vi "op_EQ_wHV.vi"(0 "Addresses Cluster":T1={"ENA1"=FALSE, "IP address 1"="172.16.14.22", "ENA2"=FALSE, "IP address 2"="172.16.14.23"}, 2 "HV parameters":T3={"Final value"=-1000, "Number of steps"=10, "Time/step"=800, "Output Off Behavior"=0, "VISA resource name"="GPIB1::25::INSTR"} {"Output Off Behavior" items=["Normal", "High Impedance", "Zero", "Guard"]; "Time/step" min=100 max=2000 step=100; "Final value" min=-1100 max=0 step=10; "Number of steps" min=10 max=20 step=10}, 3 "HV level Refnum":refnum<vi>, 4 "HV string Refnum":refnum<vi>, 5 "error tick Refnum":refnum<vi>, 6 "Operation text Refnum":refnum<vi>, 7 "EQ timeout auto Refnum":refnum<vi>, 8 "EQ wHV step barra Refnum":refnum<vi>, 9 "etapa# terminals refnums":T2, 10 "Busy Refnum":refnum<vi>, 11 "EQ steps":bool, 12 "notifier crono/Ileak":refnum<notifier>, 13 "Stop subVI Refnum":refnum<vi>) -> (15 "Folder path: equalization reports":path=path "C:/VIP Module/Files/Equalization/yyyymmdd_hh-mm-ss_Leak#_HV#", 18 "IDs summary":string, 19 "EQ summary":string)   [LabVIEW 2015, in "VIPM2.lvlib"]
doc: "Uses Notifier for Start/Stop/Exit Crono per ordres separades.\nbusy = F while waiting times and HV ramps."
uses:
  VIPM2.lvlib
panel:
  out "quants Layer":i32
  out "Chip ID list 1i2":u32[](array[numeric]) format="%.0x"
  out "I Leak":u8=3 max=3 step=1
  out "Global Reg (hex)":u32[](array[numeric])=[68228136, 235670073, 4294967264, 4294967295, 4294967295, 511] format="%x"
  out "PixelReg (hex)":u32[](array[numeric])=[671965161, 384, 671965161, 384, 671965161, 384, 671965161, 384, 671965161, 384, 671965161, 384, 671965161, 384, 671965161, 384, 671965161, 384, 671965161, 384, 671965161, 384, 671965161, 384, 671965161, 384, 671965161, 384, 671965161, 384, 671965161, 384, 671965161, 384, 671965161, 384, 671965161, 384, 671965161, 384, 671965161, 384, 671965161, 384, 671965161, 384, 671965161, 384, 671965161, 384, 671965161, 384, 671965161, 384, 671965161, 384, 671965161, 384, 671965161, 384, 671965161, 384, 671965161, 384, 671965161, 384, 671965161, 384, 671965161, 384, 671965161, 384, 671965161, 384, 671965161, 384, 671965161, 384, 671965161, 384, 671965161, 384, 671965161, 384, 671965161, 384, 671965161, 384, 671965161, 384, 671965161, 384, 671965161, 384, 671965161, 384, 671965161, 384, 671965161, 384, 671965161, 384, 671965161, 384, 671965161, 384, 671965161, 384, 671965161, 384, 671965161, 384, 671965161, 384, 671965161, 384, 671965161, 384, 671965161, 384, 671965161, 384, 671965161, 384, 671965161, 384, 671965161, 384, 671965161, 384, 671965161, 384, 671965161, 384, 671965161, 384, 671965161, 384, 671965161, 384, 671965161, 384, 671965161, 384, 671965161, 384, 671965161, 384, 671965161, 384, 671965161, 384, 671965161, 384, 671965161, 384, 671965161, 384, 671965161, 384, 671965161, 384, 671965161, 384, 671965161, 384, 671965161, 384, 671965161, 384, 671965161, 384, 671965161, 384, 671965161, 384, 671965161, 384, 671965161, 384, 671965161, 384, 671965161, 384, 671965161, 384, 671965161, 384, 671965161, 384, 671965161, 384, 671965161, 384, 671965161, 384, 671965161, 384, 671965161, 384] format="%x"
  in  "EQ parameters (cluster)":T4={"Timeout ITEST sweep"=21, "Number pulses ITEST"=20, "TOT"=40, "ADC target"=900, "Number pulses SSpeak sweep"=100, "Timeout SSpeak sweep"=110, "Timeout THLD sweep"=10, "Number triggers THLD sweep"=2, "First PIXEL"=0, "Last PIXEL"=99, "Sigma factor"=2, "DTP period for SSpeak sweep"=1, "Global THR for ITEST sweep"=38, "Pulse width"=0} {"Number triggers THLD sweep" step=1; "Timeout THLD sweep" step=1; "Timeout SSpeak sweep" step=1; "DTP period for SSpeak sweep" step=1; "Number pulses SSpeak sweep" step=1; "Timeout ITEST sweep" step=1; "Global THR for ITEST sweep" step=1; "Number pulses ITEST" step=1; "Pulse width" items=["25 ns", "50 ns", "75 ns", "100 ns"]; "Sigma factor" step=1; "Last PIXEL" max=99 step=1; "First PIXEL" max=99 step=1; "ADC target" step=1; "TOT" step=1}
  # "Operation: EQualization with HV (refnums)"
  # "Uses Notifier for\nStart/Stop/Exit Crono"
  # "I test sweep"
  # "SS peak sweep"
  # "THLD sweep"
  # "Number of triggers"
  # "Timeout"
  # "Timeout"
  # "DTP period"
  # "Number of pulses"
  # "Timeout"
  # "Global THR"
  # "Number of pulses"
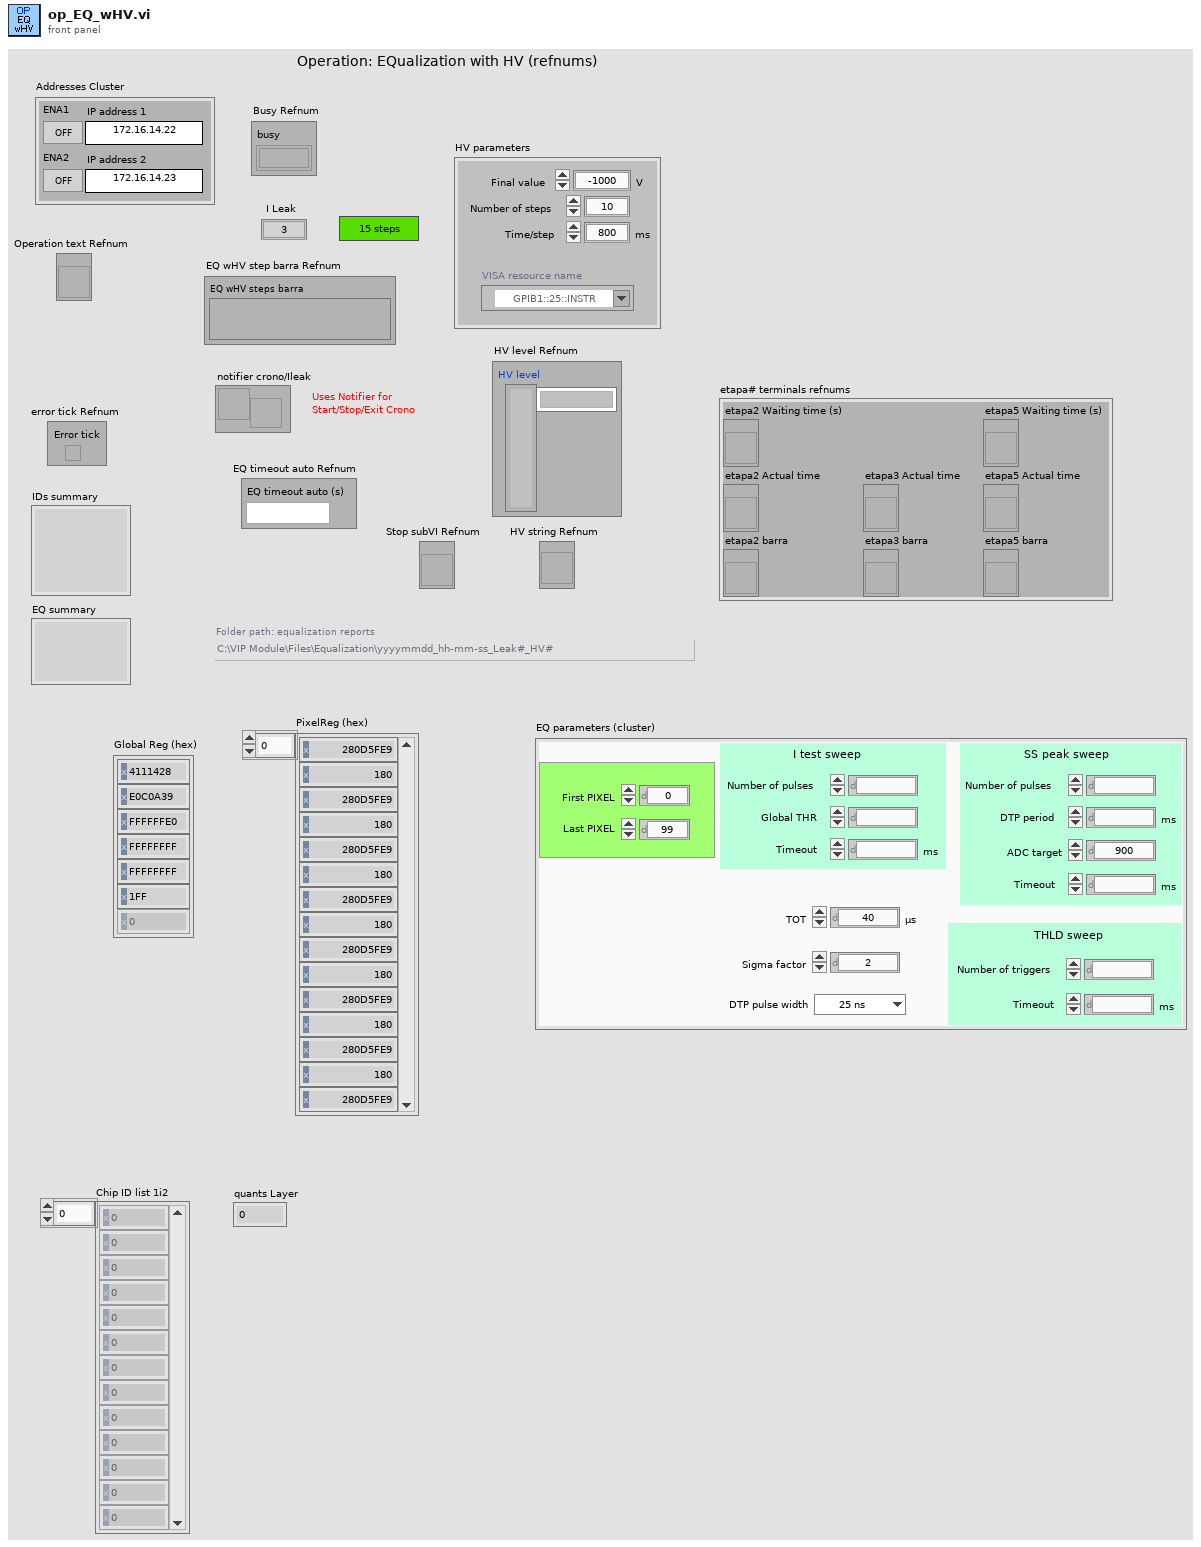
[diagram p1: front panel]
types:
  T1 = cluster{"ENA1":bool, "IP address 1":string, "ENA2":bool, "IP address 2":string}
  T2 = cluster{"etapa2 Waiting time (s)":refnum<vi>, "etapa2 Actual time":refnum<vi>, "etapa2 barra":refnum<vi>, "etapa3 Actual time":refnum<vi>, "etapa3 barra":refnum<vi>, "etapa5 Waiting time (s)":refnum<vi>, "etapa5 Actual time":refnum<vi>, "etapa5 barra":refnum<vi>}
  T3 = cluster{"Final value":i16, "Number of steps":u8, "Time/step":u16, "Output Off Behavior":u16, "VISA resource name":refnum<visa-resource-name>}
  T4 = cluster{"Timeout ITEST sweep":u32, "Number pulses ITEST":u32, "TOT":u32, "ADC target":u32, "Number pulses SSpeak sweep":u32, "Timeout SSpeak sweep":u32, "Timeout THLD sweep":u32, "Number triggers THLD sweep":u32, "First PIXEL":u32, "Last PIXEL":u32, "Sigma factor":u32, "DTP period for SSpeak sweep":u32, "Global THR for ITEST sweep":u32, "Pulse width":u32}
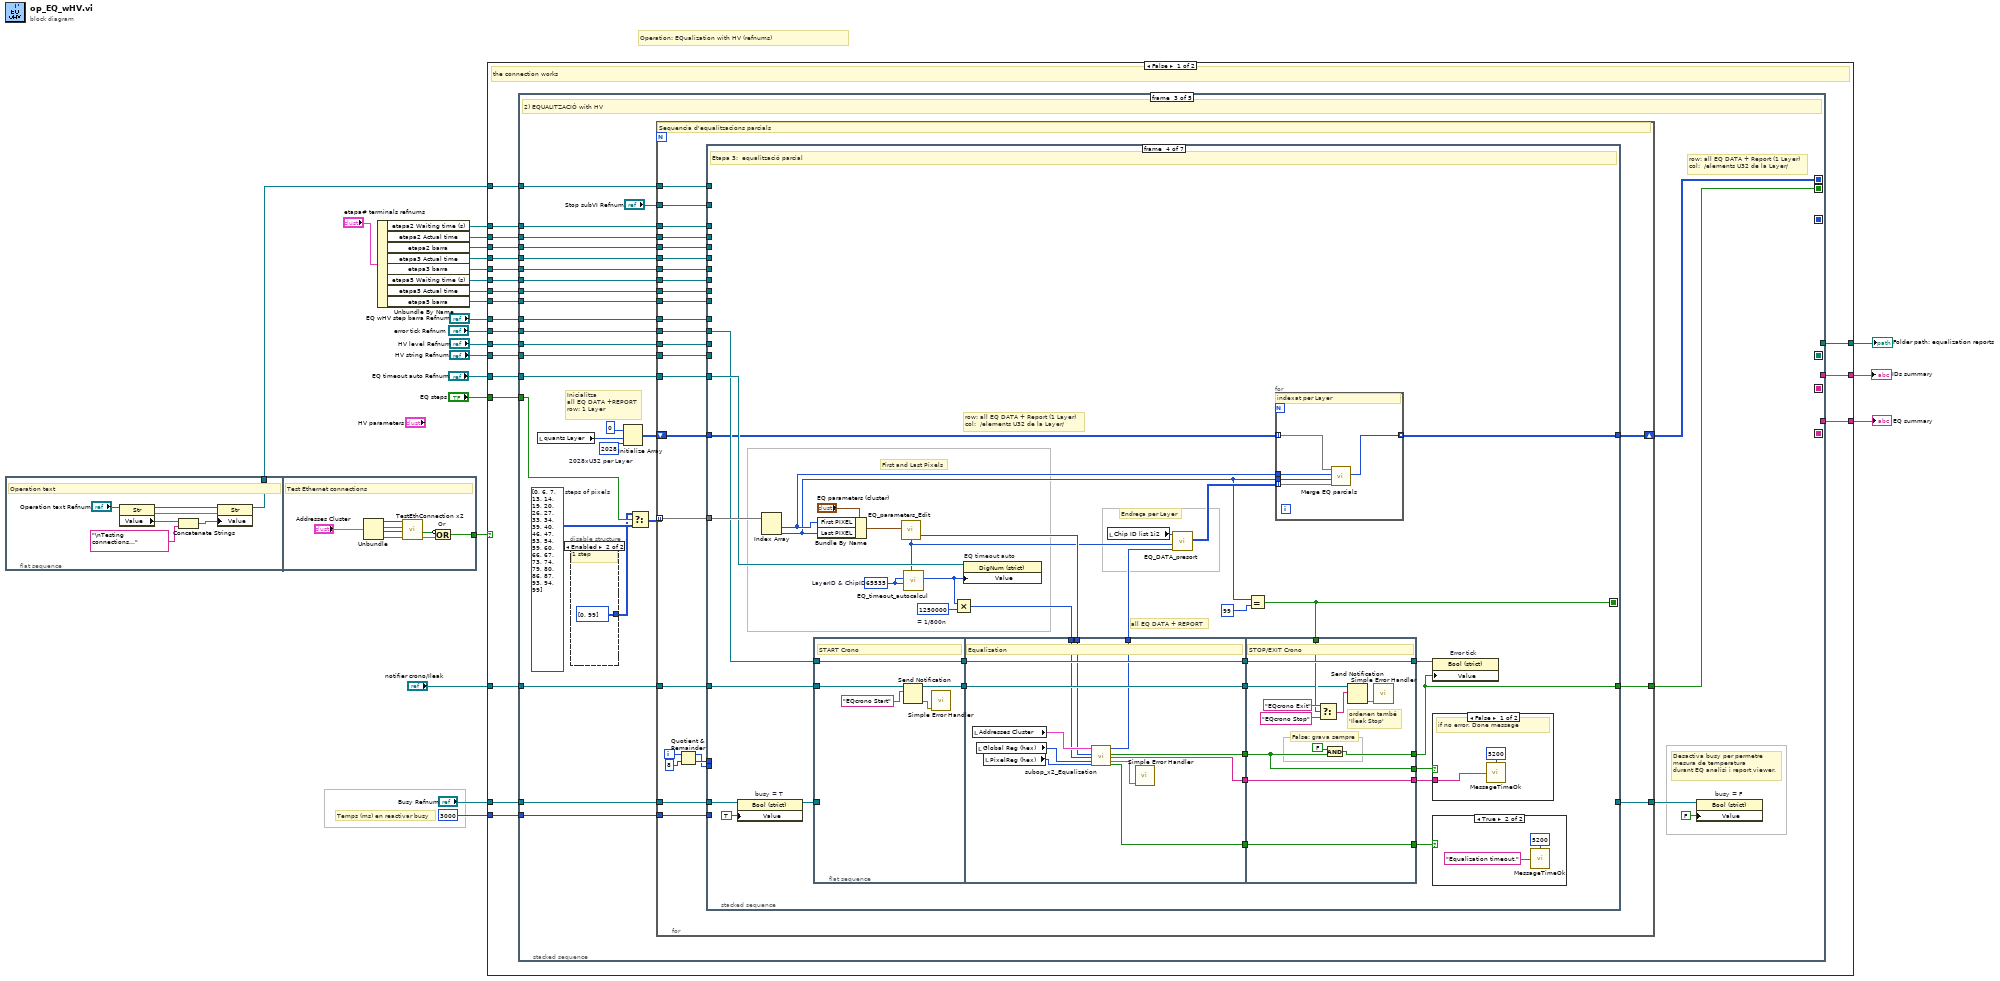
[diagram p0: block diagram]
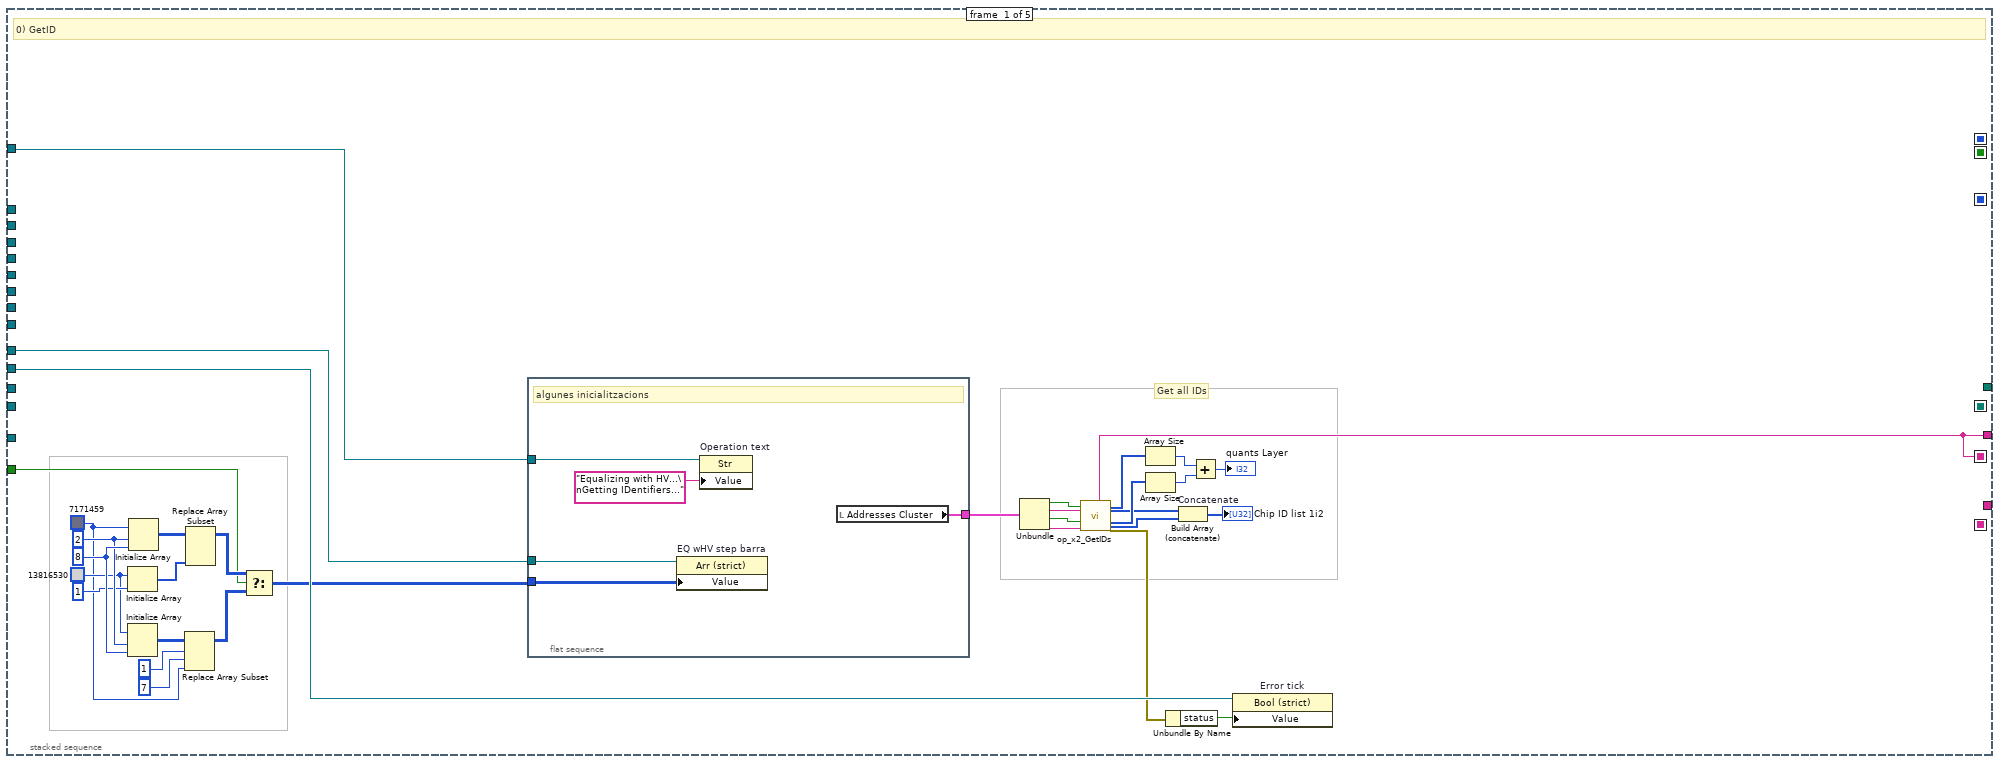
[diagram p2: hidden frame]
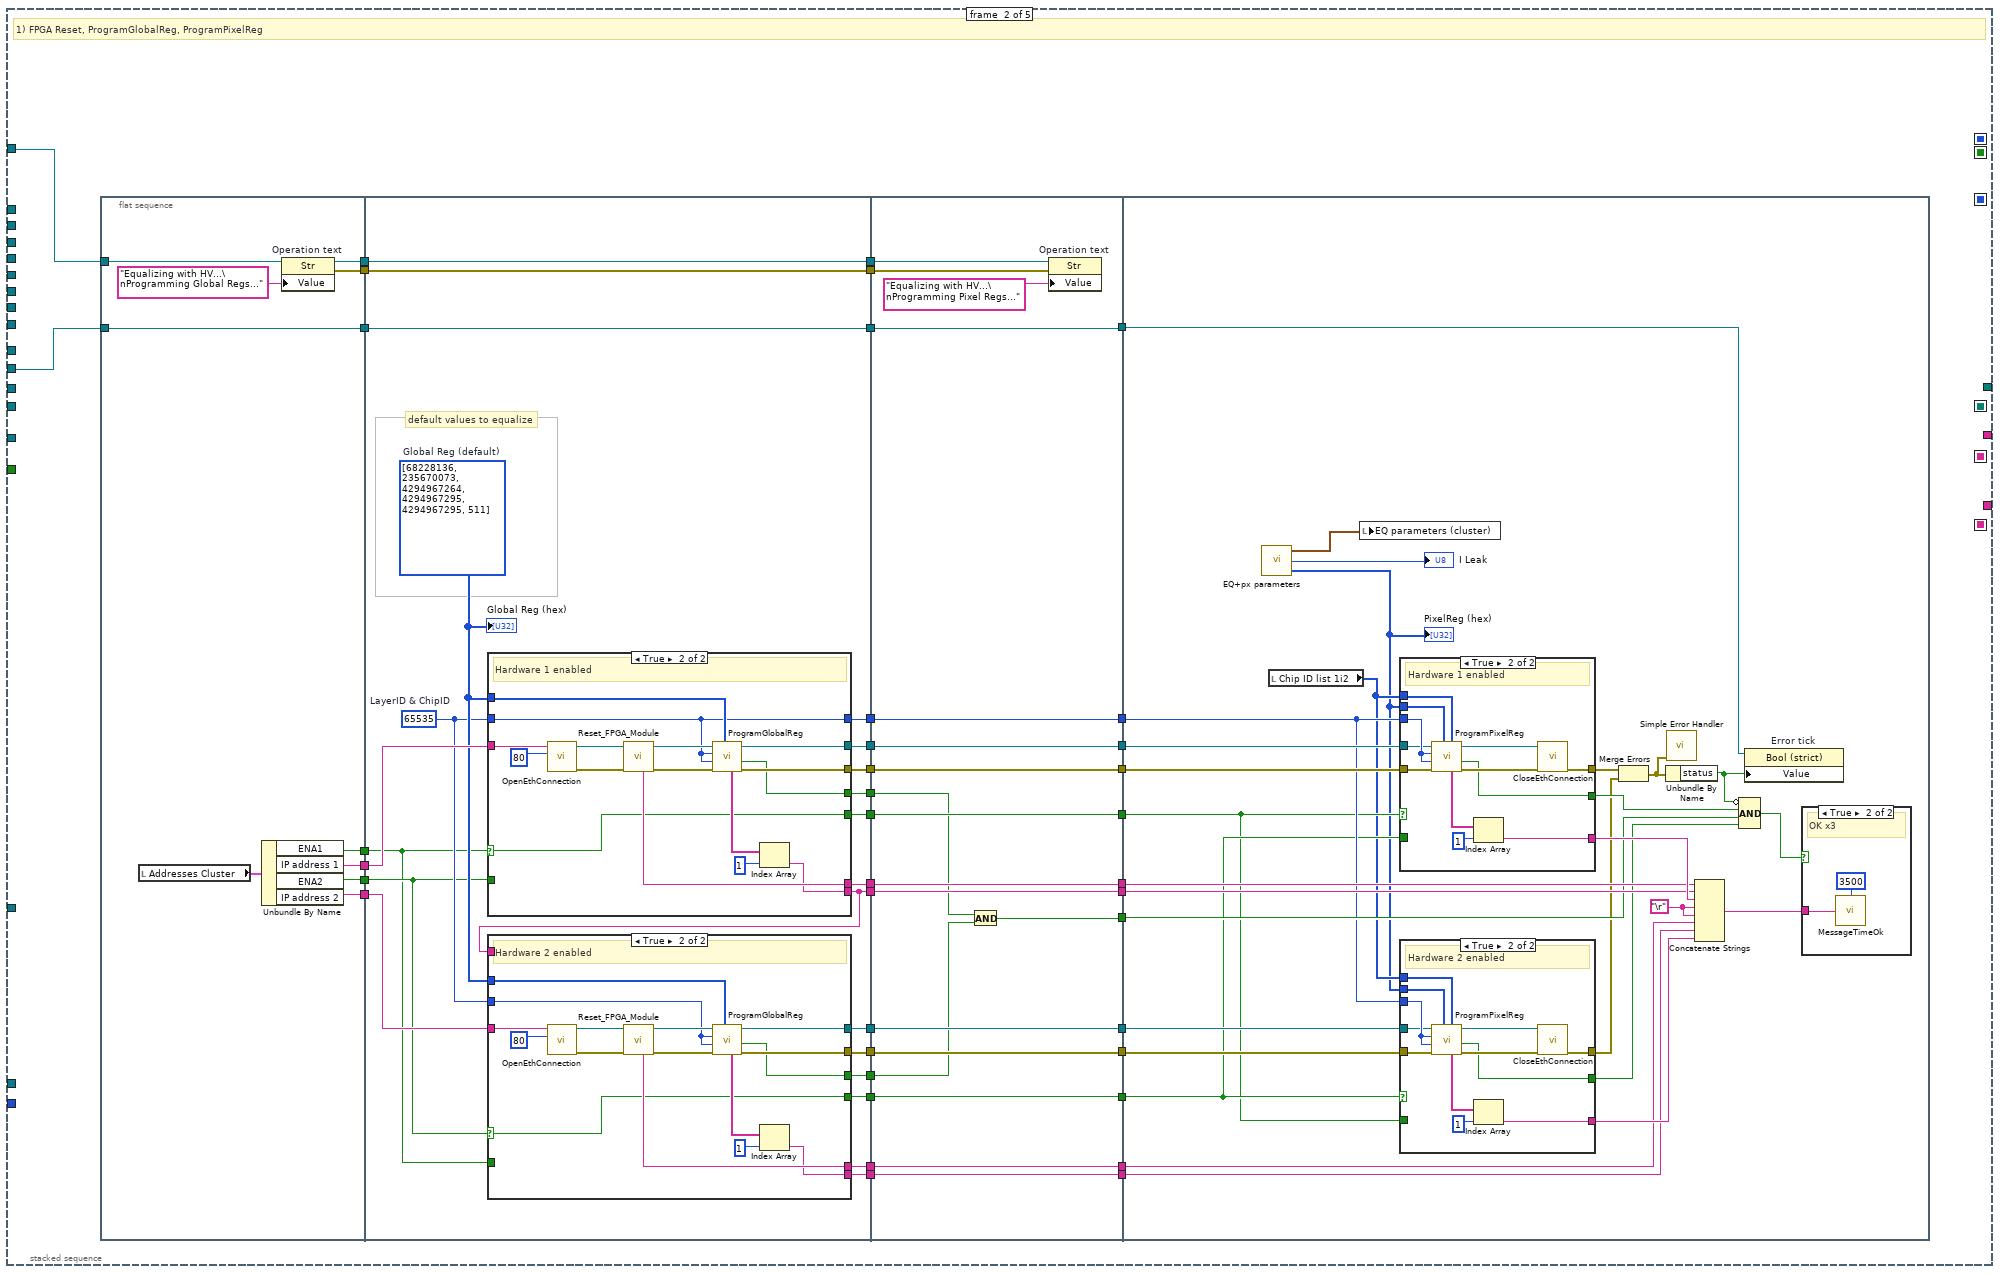
[diagram p3: hidden frame]
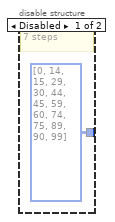
[diagram p9: hidden frame]
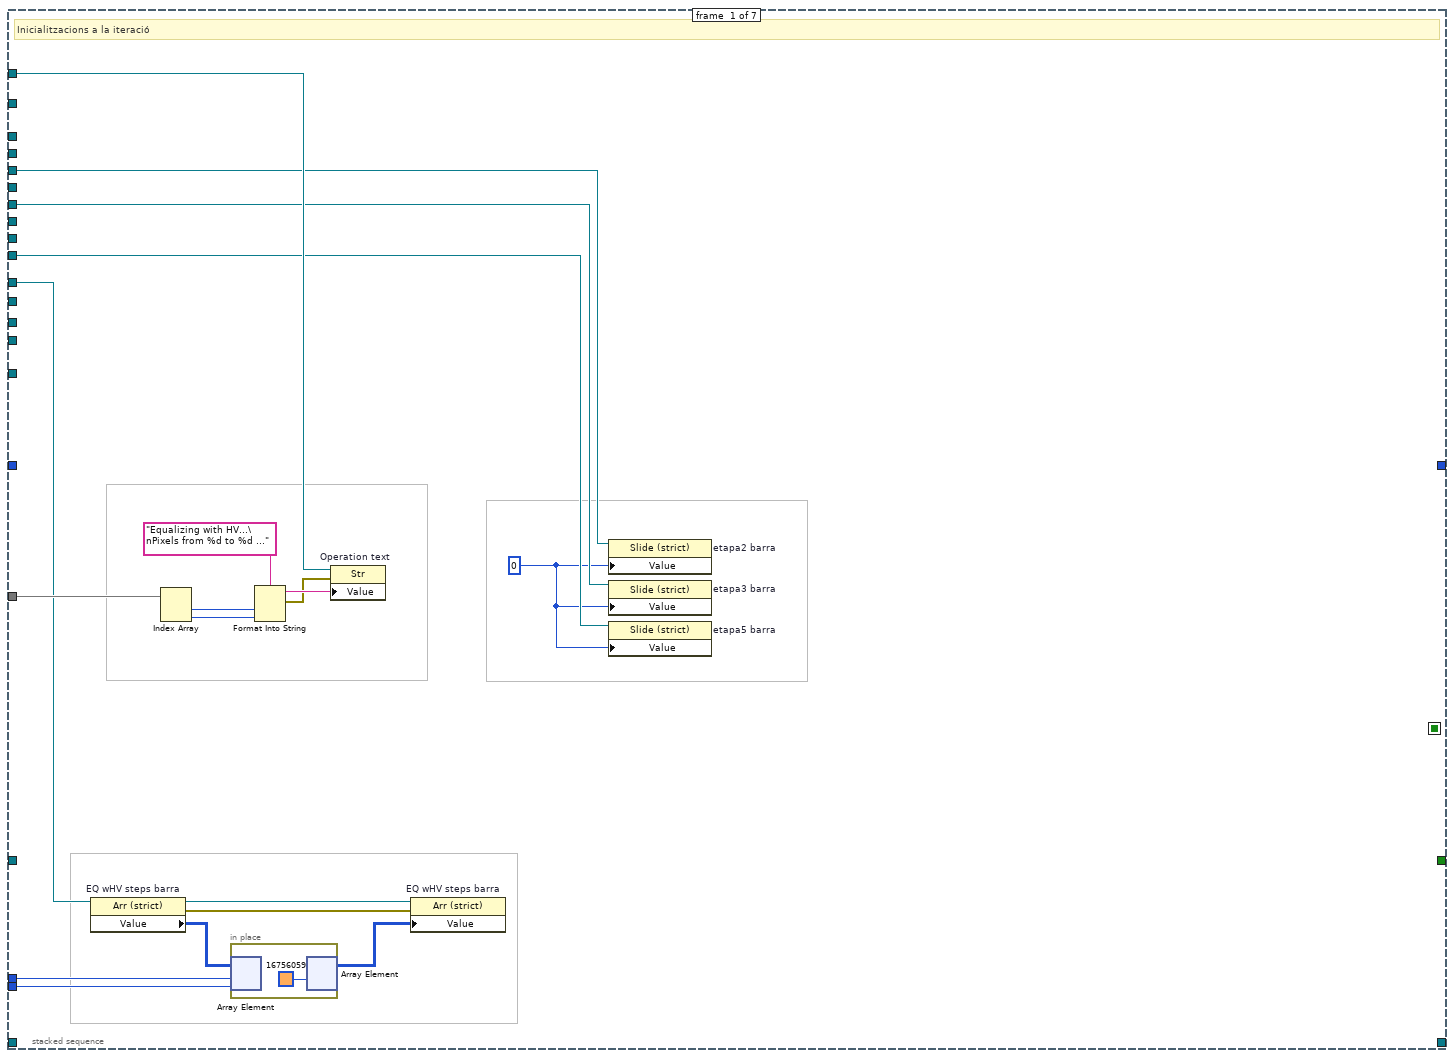
[diagram p10: hidden frame]
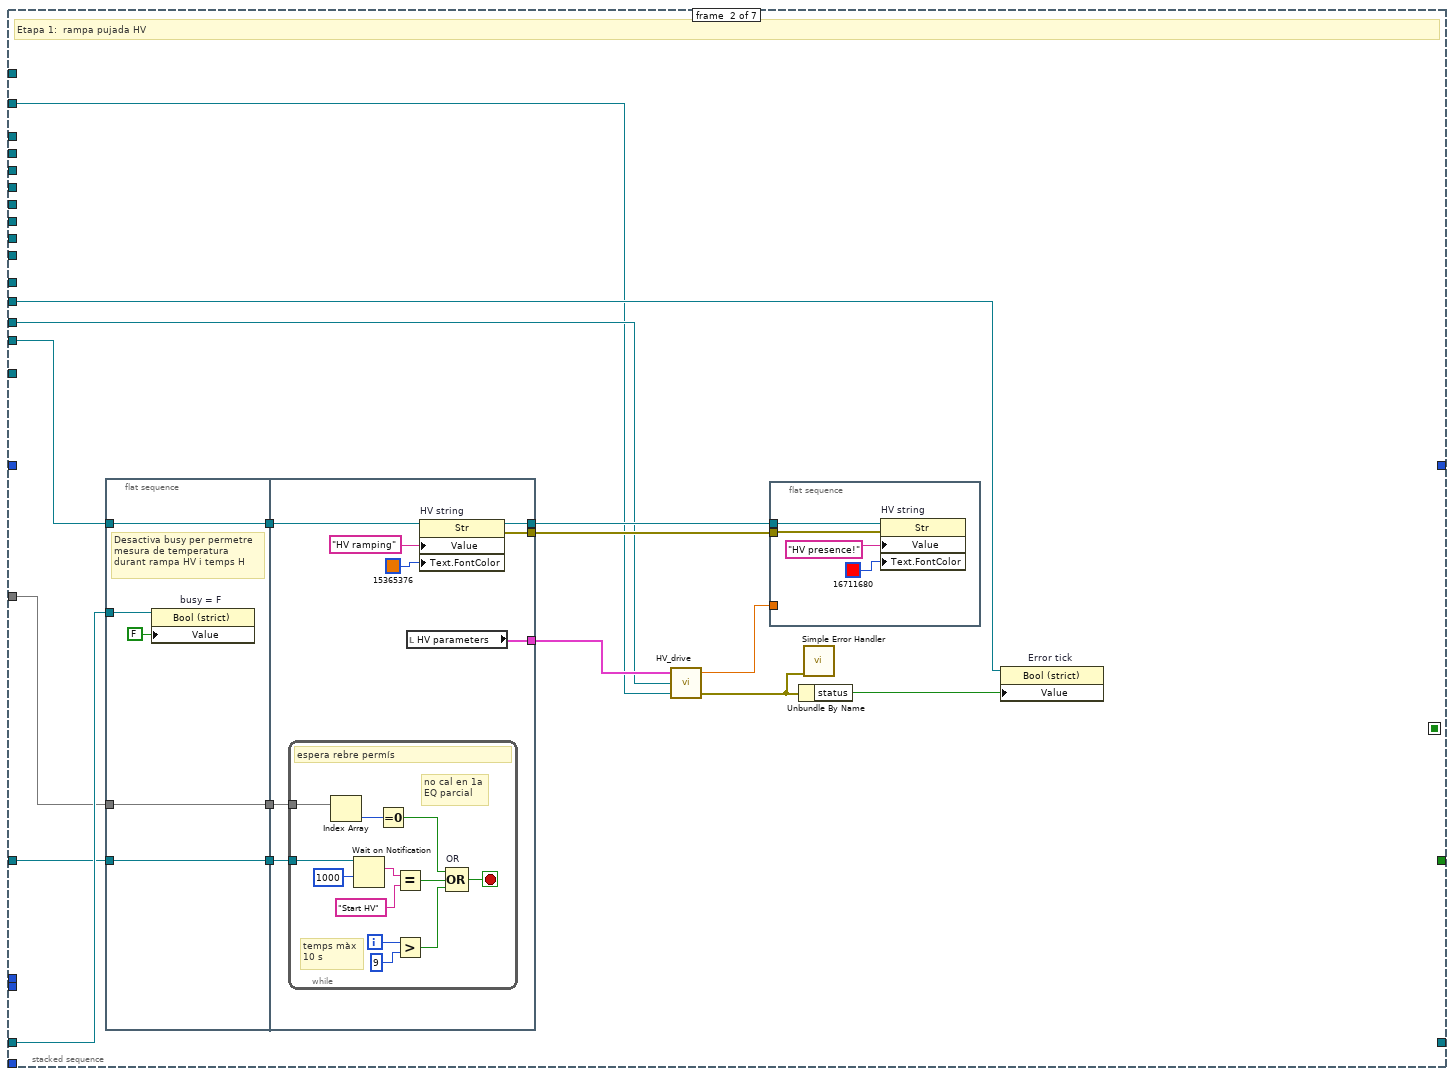
[diagram p11: hidden frame]
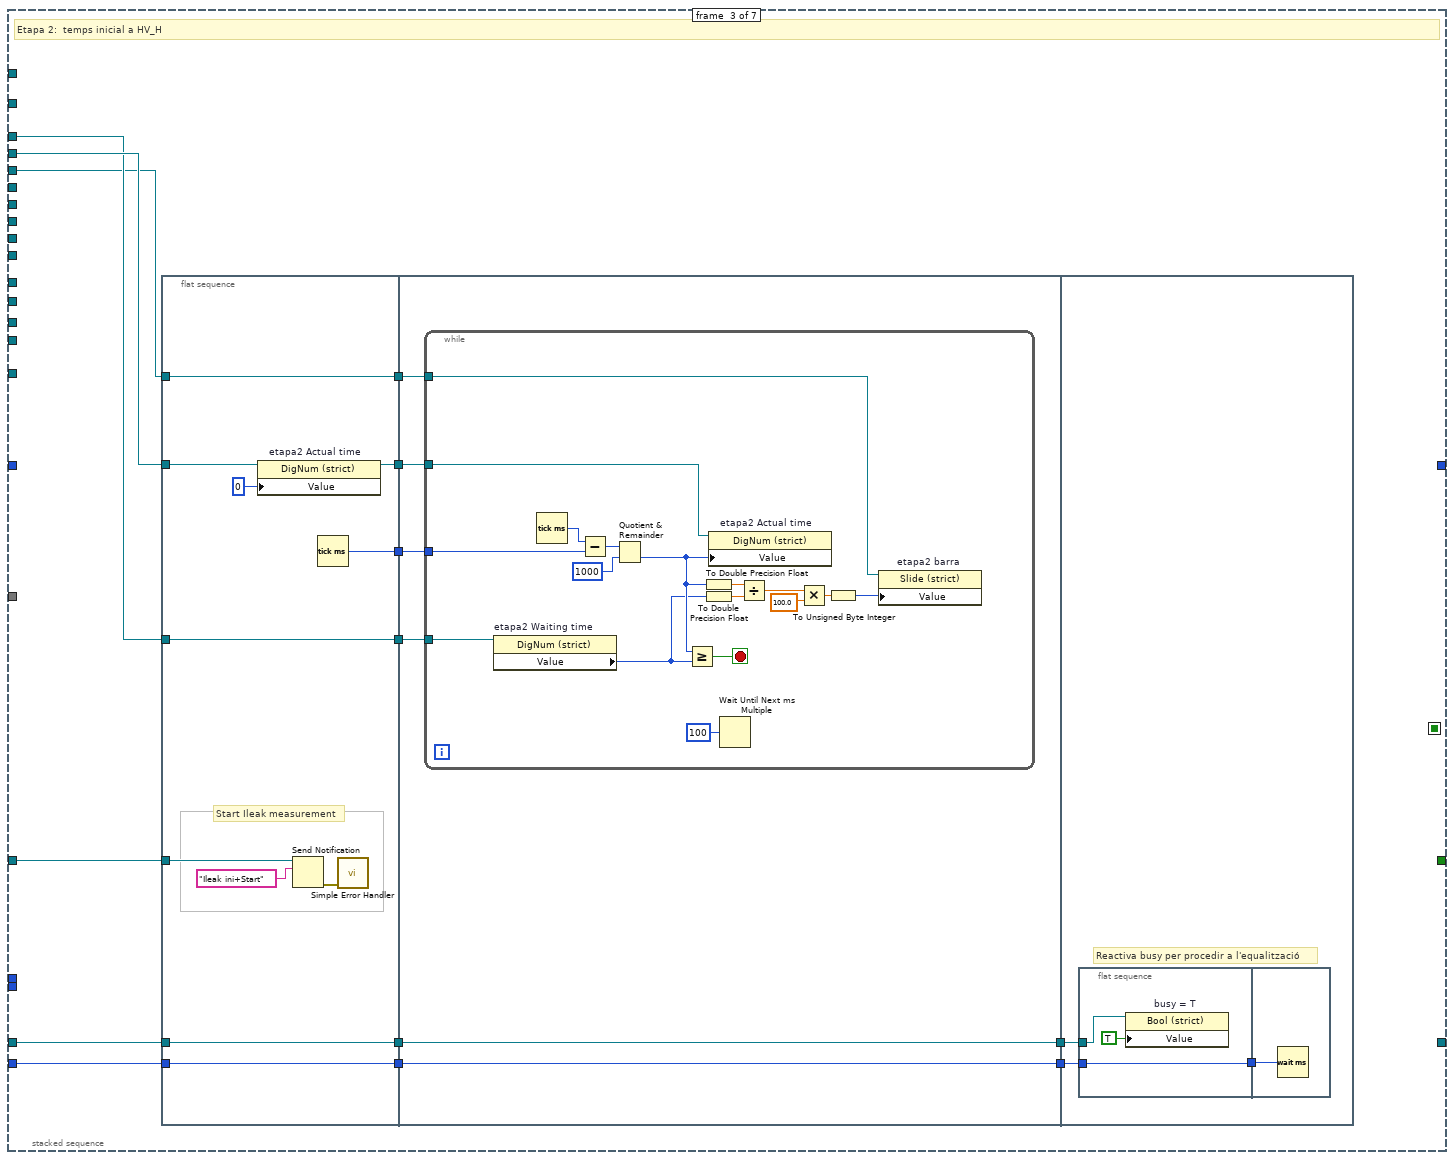
[diagram p12: hidden frame]
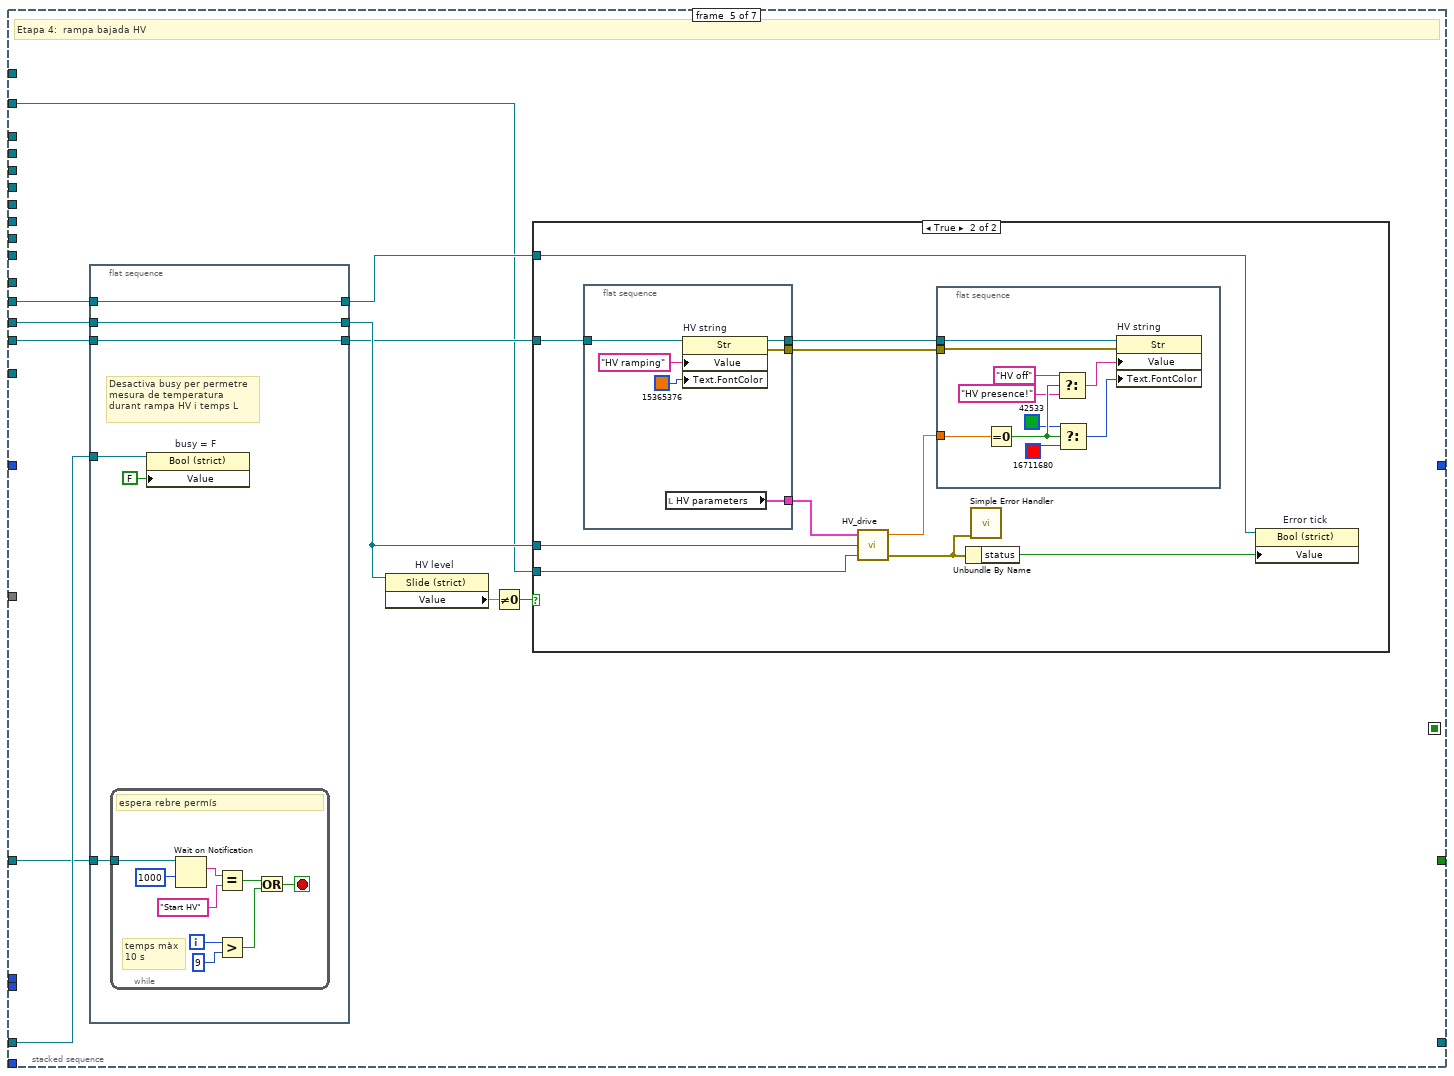
[diagram p15: hidden frame]
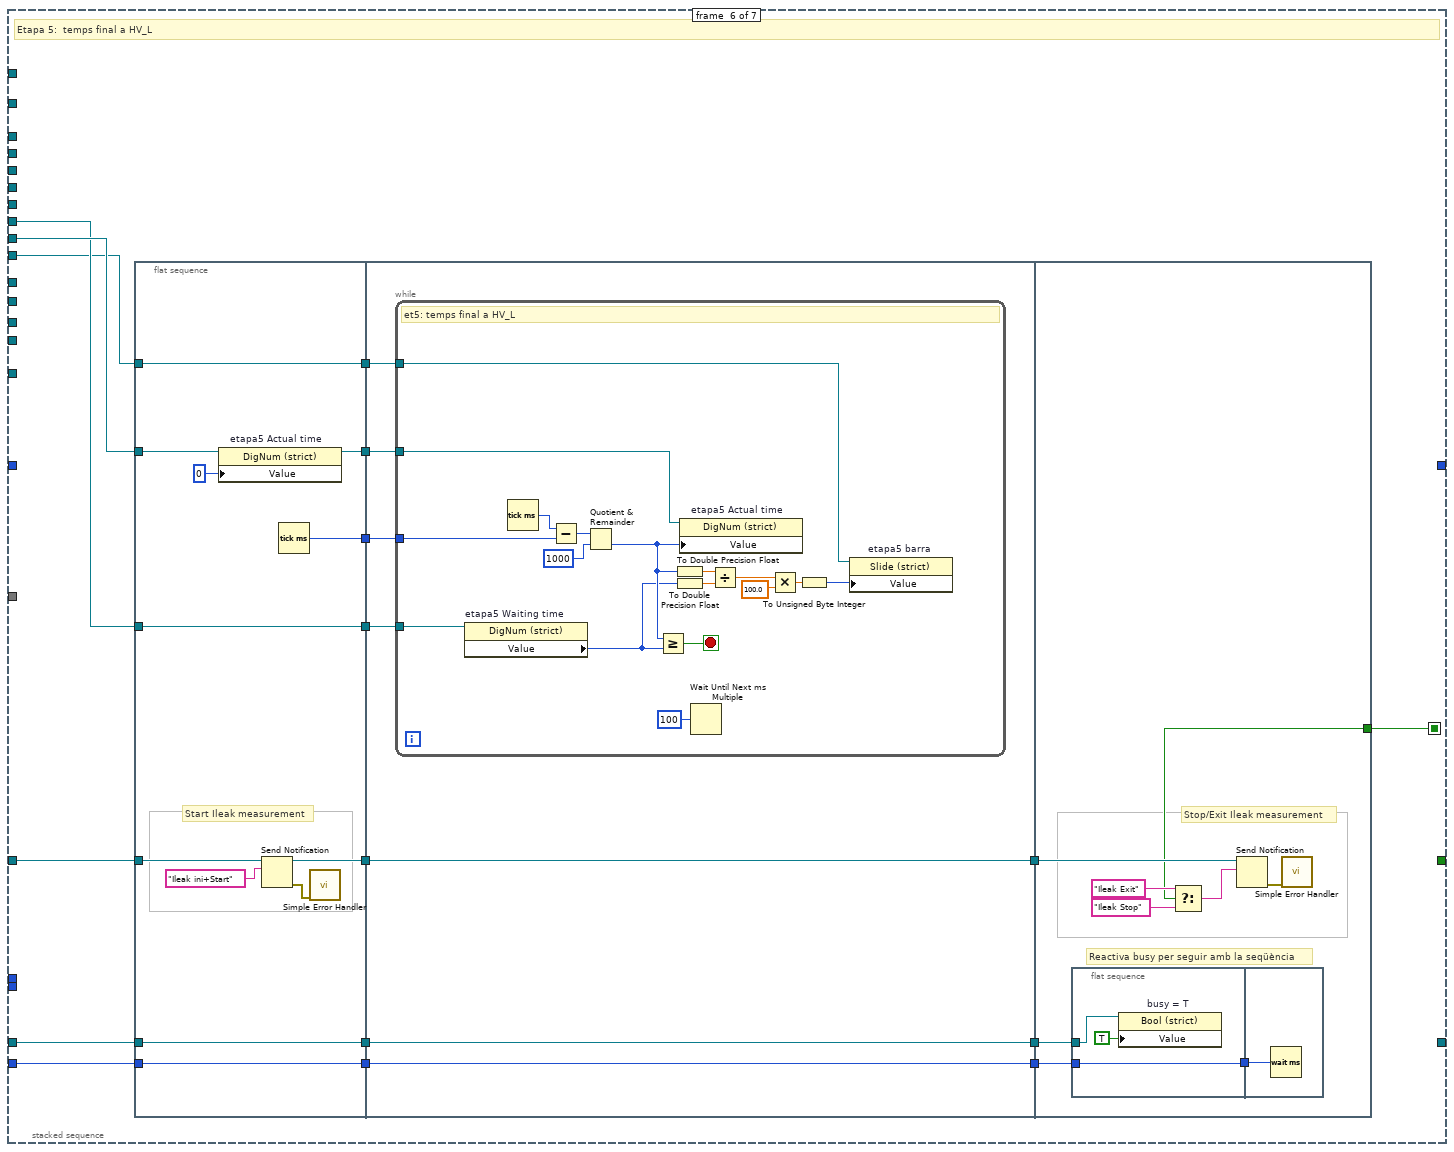
[diagram p17: hidden frame]
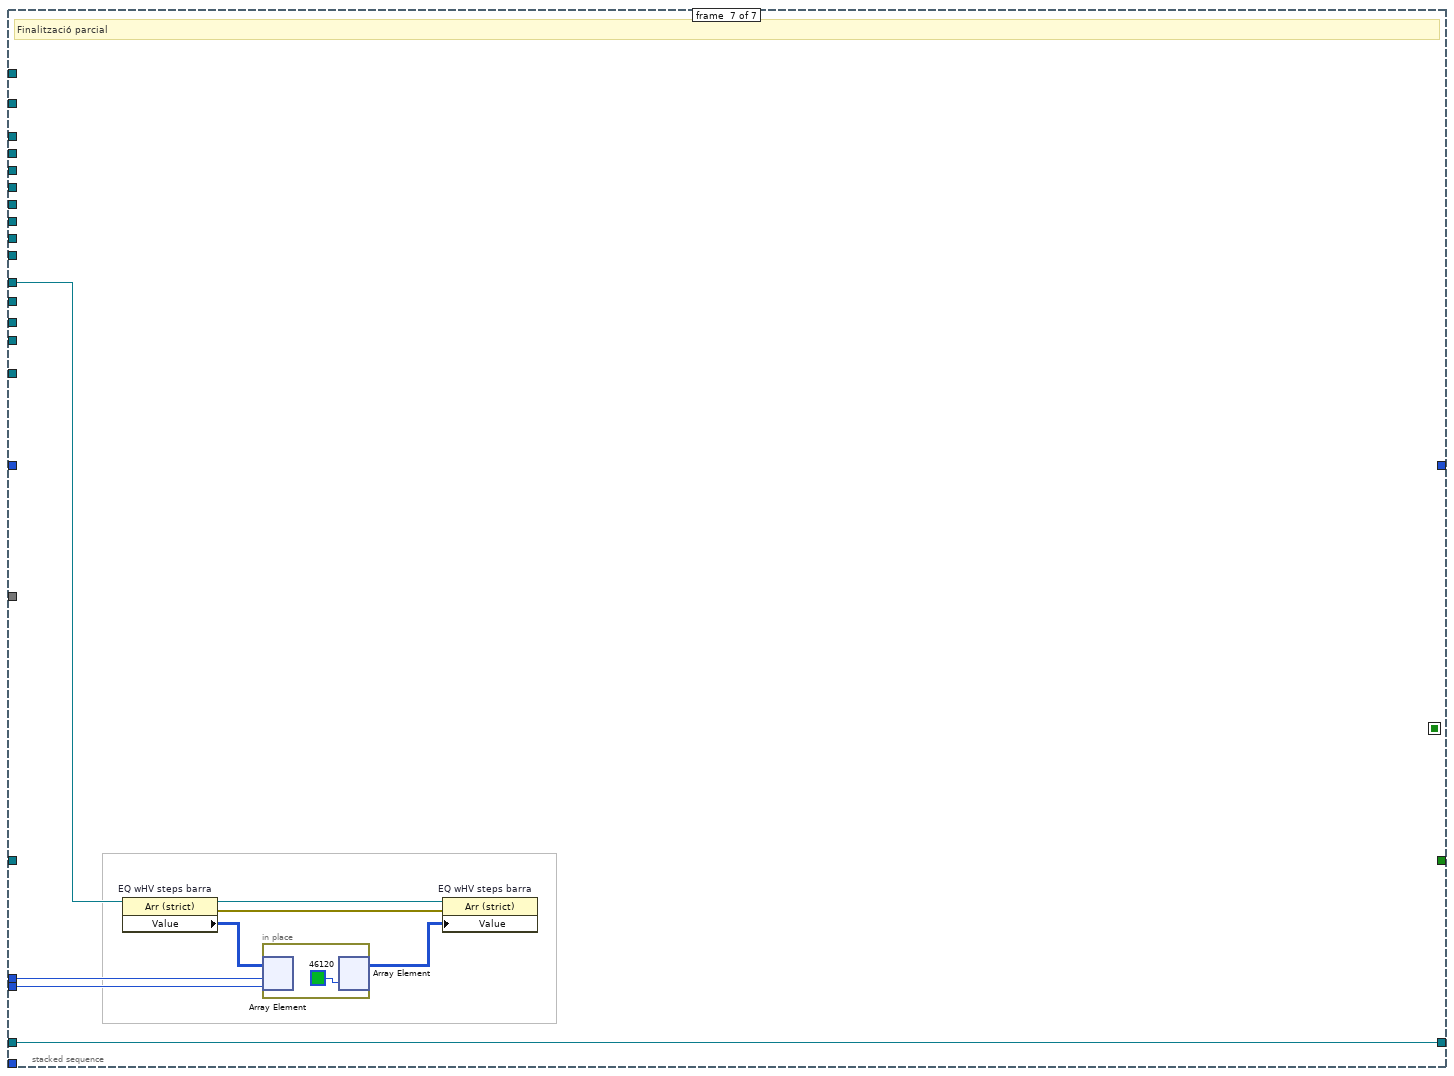
[diagram p18: hidden frame]
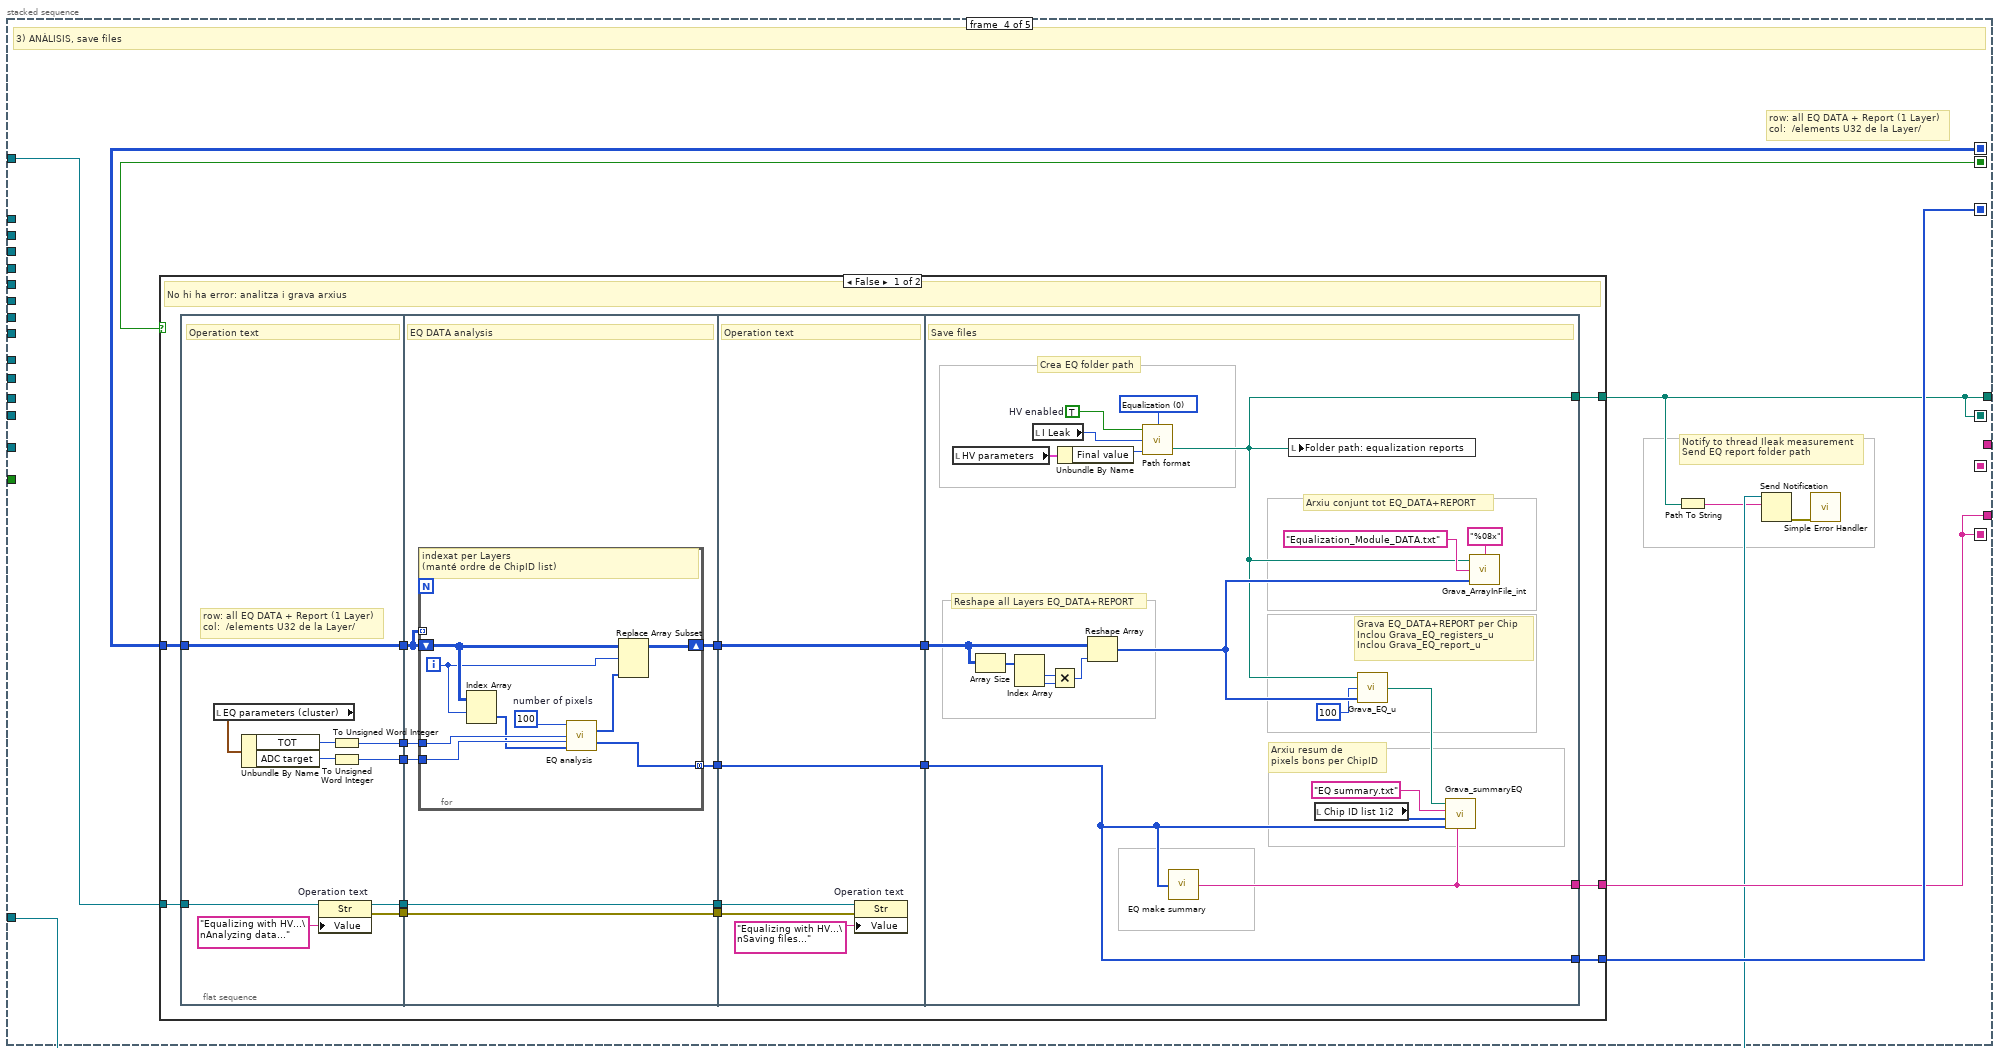
[diagram p19: hidden frame]
diagram:
  # "Temps (ms) en reactivar busy"
  # "Operation: EQualization with HV (refnums)"
  n1 = flat-sequence {
    tunnel: [w24] -> w13
    tunnel: [w38] -> w23
    frame #0 {
      # "Operation text"
      n2 = property class="Str"(reference="Operation text Refnum") -> (reference out=w27:refnum<vi>, error out=w26:errorcluster, "Value"=w29:string)  [unwired: 1 in]
      n3 = Concatenate Strings "Concatenate Strings"(w29, "\nTesting connections..." ("string")) -> (w25:string)
      n4 = property class="Str"(reference=w27, error in=w26, "Value"=w25) -> (reference out=w24:refnum<vi>)  [unwired: 1 out]
    }
    frame #1 {
      # "Test Ethernet connections"
      n5 = Unbundle("Addresses Cluster") -> ("ENA1"=w34:bool, "IP address 1"=w33:string, "ENA2"=w32:bool, "IP address 2"=w31:string)
      n6 = call "TestEthConnection x2.vi"("IP address 2"=w31, "ENA2"=w32, "IP address 1"=w33, "ENA1"=w34) -> ("error out"=w36:errorcluster, "Answers OK?"=w37:bool)  [unwired: 6 in]
      n7 = Compound Arithmetic op=OR "Or"(invert w37, w36) -> (w38:bool)
    }
  }
  n8 = Unbundle By Name("etapa# terminals refnums") -> ("etapa2 Waiting time (s)"=w21:refnum<vi>, "etapa2 Actual time"=w20:refnum<vi>, "etapa2 barra"=w19:refnum<vi>, "etapa3 Actual time"=w18:refnum<vi>, "etapa3 barra"=w17:refnum<vi>, "etapa5 Waiting time (s)"=w16:refnum<vi>, "etapa5 Actual time"=w15:refnum<vi>, "etapa5 barra"=w14:refnum<vi>)
  n9 = case shown="False" w23 {
    selector: w23 -> [_ w763]
    tunnel: w21 -> [w58 _]
    tunnel: w20 -> [w57 _]
    tunnel: w19 -> [w56 _]
    tunnel: w18 -> [w55 _]
    tunnel: w17 -> [w54 _]
    tunnel: w16 -> [w53 _]
    tunnel: w15 -> [w52 _]
    tunnel: w14 -> [w51 _]
    tunnel: w13 -> [w59 _]
    tunnel: "EQ wHV step barra Refnum" -> [w50 _]
    tunnel: "HV level Refnum" -> [w48 _]
    tunnel: "HV string Refnum" -> [w47 _]
    tunnel: "EQ timeout auto Refnum" -> [w46 _]
    tunnel: "error tick Refnum" -> [w49 w762]
    tunnel: [w44 _] -> w7
    tunnel: [w45 _] -> w6
    tunnel: [w43 _] -> w5
    tunnel: "notifier crono/Ileak" -> [w42 _]
    tunnel: "Busy Refnum" -> [w41 _]
    tunnel: u32 3000 -> [w40 _]
    tunnel: "EQ steps" -> [w39 _]
    frame False {
      # "the connection works"
      n10 = stacked-sequence {
        seq-local: [_ _ w308 _ _] -> [_ _ _ w667 _]
        seq-local: [_ _ w294 _ _] -> [_ _ _ w668 w741]
        seq-local: [_ _ _ w665 _] -> [_ _ _ _ w740]
        seq-local: [w82 _ _ _ _] -> [_ _ _ _ w739]
        seq-local: [_ _ _ w664 _] -> [_ _ _ _ w738]
        seq-local: [_ _ _ w660 _] -> [_ _ _ _ w736]
        tunnel: w59 -> [w92 w135 w307 w666 w737]
        tunnel: w58 -> [_ _ w306 _ _]
        tunnel: w57 -> [_ _ w305 _ _]
        tunnel: w56 -> [_ _ w304 _ _]
        tunnel: w55 -> [_ _ w303 _ _]
        tunnel: w54 -> [_ _ w302 _ _]
        tunnel: w53 -> [_ _ w301 _ _]
        tunnel: w52 -> [_ _ w300 _ _]
        tunnel: w51 -> [_ _ w299 _ _]
        tunnel: w50 -> [w91 _ w298 _ _]
        tunnel: w49 -> [w90 w115 w295 _ _]
        tunnel: w48 -> [_ _ w297 _ _]
        tunnel: w47 -> [_ _ w296 _ _]
        tunnel: w46 -> [_ _ w293 _ _]
        tunnel: [w82 _ _ _ _] -> w45
        tunnel: [_ _ _ w660 _] -> w44
        tunnel: [_ _ _ w664 _] -> w43
        tunnel: w42 -> [_ _ w290 w662 _]
        tunnel: w41 -> [_ _ w289 _ _]
        tunnel: w40 -> [_ _ w288 _ _]
        tunnel: w39 -> [w61 _ w284 _ _]
        frame #0 {
          w67 = u32 13816530
          w73 = 8 ("dimension size")
          w63 = u32 7171459
          w72 = 2 ("dimension size")
          # "Get all IDs"
          # "0) GetID"
          n11 = Initialize Array(w67, 1 ("dimension size")) -> (w65:u32[])
          n12 = Initialize Array "Initialize Array"(w67, w72, w73) -> (w66:u32[][])
          n13 = Initialize Array "Initialize Array"(w63, w72, w73) -> (w64:u32[][])
          n14 = Replace Array Subset(array=w66, new element=w63, index (row)=1, index (col)=7 ("index (row)")) -> (w71:u32[][])
          n15 = Replace Array Subset(array=w64, new element=w65) -> (w70:u32[][])  [unwired: 2 in]
          n16 = Select(t=w70, s=w61, f=w71) -> (s? t:f=w60:u32[][])
          n17 = flat-sequence {
            tunnel: [w97] -> w87
            tunnel: w92 -> [w96]
            tunnel: w91 -> [w94]
            tunnel: w60 -> [w93]
            frame #0 {
              # "algunes inicialitzacions"
              n18 = property on="EQ wHV step barra" class="Arr (strict)"(reference=w94, "Value"=w93) -> ()  [unwired: 1 in, 2 out]
              n19 = property on="Operation text" class="Str"(reference=w96, "Value"="Equalizing with HV...\nGetting IDentifiers...") -> ()  [unwired: 1 in, 2 out]
              n20 = local read "Addresses Cluster"() -> (w97:T1)
            }
          }
          n21 = Unbundle(w87) -> ("ENA1"=w86:bool, "IP address 1"=w85:string, "ENA2"=w84:bool, "IP address 2"=w83:string)
          n22 = call "op_x2_GetIDs.vi"("ENA1"=w86, "IP address 1"=w85, "ENA2"=w84, "IP address 2"=w83) -> ("summary IDs"=w82:string, "Layer ID list 1 (ordered)"=w78:u32[], "Chip ID list 1"=w76:u32[], "Layer ID list 2 (ordered)"=w77:u32[], "Chip ID list 2"=w75:u32[], "error out"=w88:errorcluster)  [unwired: 16 in, 2 out]
          n23 = Array Size(array=w78) -> (size(s)=w80:i32)
          n24 = Array Size(array=w77) -> (size(s)=w79:i32)
          n25 = Unbundle By Name(w88) -> ("status"=w89:bool)
          n26 = Build Array (concatenate) "Concatenate"(w76, w75) -> (→"Chip ID list 1i2":u32[])
          n27 = Add(x=w80, y=w79) -> (x+y=→"quants Layer":i32)
          n28 = property on="Error tick" class="Bool (strict)"(reference=w90, "Value"=w89) -> ()  [unwired: 1 in, 2 out]
        }
        frame #1 {
          # "1) FPGA Reset, ProgramGlobalReg, ProgramPixelReg"
          n29 = flat-sequence {
            tunnel: w135 -> [w144]
            tunnel: [w143] -> w134
            tunnel: [w142] -> w133
            tunnel: [w141] -> w116
            tunnel: w115 -> [w141]
            tunnel: [w139] -> w112
            tunnel: [w138] -> w111
            tunnel: [w137] -> w110
            tunnel: [w136] -> w109
            tunnel: w134 -> [w167]
            tunnel: w133 -> [w166]
            tunnel: [w167] -> w132
            tunnel: [w166] -> w131
            tunnel: [w160] -> w129
            tunnel: [w165] -> w127
            tunnel: [w164] -> w125
            tunnel: [w163] -> w123
            tunnel: [w146] -> w121
            tunnel: [w162] -> w119
            tunnel: [w161] -> w117
            tunnel: w116 -> [w161]
            tunnel: [w159] -> w114
            tunnel: w112 -> [w153]
            tunnel: w111 -> [w158]
            tunnel: w110 -> [w154]
            tunnel: w109 -> [w155]
            tunnel: [w152] -> w107
            tunnel: [w151] -> w105
            tunnel: [w150] -> w103
            tunnel: [w149] -> w102
            tunnel: [w148] -> w100
            tunnel: [w147] -> w98
            tunnel: w132 -> [w221]
            tunnel: w131 -> [w220]
            tunnel: [w219] -> w130
            tunnel: w129 -> [w219]
            tunnel: [w218] -> w128
            tunnel: w127 -> [w218]
            tunnel: [w217] -> w126
            tunnel: w125 -> [w217]
            tunnel: [w216] -> w124
            tunnel: w123 -> [w216]
            tunnel: [w215] -> w122
            tunnel: w121 -> [w215]
            tunnel: [w207] -> w120
            tunnel: w119 -> [w211]
            tunnel: [w214] -> w118
            tunnel: w117 -> [w214]
            tunnel: w114 -> [w213]
            tunnel: [w213] -> w113
            tunnel: [w212] -> w108
            tunnel: w107 -> [w212]
            tunnel: [w210] -> w106
            tunnel: w105 -> [w210]
            tunnel: [w209] -> w104
            tunnel: w103 -> [w209]
            tunnel: w102 -> [w208]
            tunnel: [w206] -> w101
            tunnel: w100 -> [w206]
            tunnel: [w205] -> w99
            tunnel: w98 -> [w205]
            tunnel: w130 -> [w239]
            tunnel: w128 -> [w247]
            tunnel: w126 -> [w246]
            tunnel: w124 -> [w245]
            tunnel: w122 -> [w244]
            tunnel: w120 -> [w243]
            tunnel: w118 -> [w242]
            tunnel: w113 -> [w235]
            tunnel: w108 -> [w238]
            tunnel: w106 -> [w237]
            tunnel: w104 -> [w236]
            tunnel: w101 -> [w228]
            tunnel: w99 -> [w229]
            frame #0 {
              n30 = local read "Addresses Cluster"() -> (w140:T1)
              n31 = Unbundle By Name(w140) -> ("ENA1"=w139:bool, "IP address 1"=w138:string, "ENA2"=w137:bool, "IP address 2"=w136:string)
              n32 = property on="Operation text" class="Str"(reference=w144, "Value"="Equalizing with HV...\nProgramming Global Regs...") -> (reference out=w143:refnum<vi>, error out=w142:errorcluster)  [unwired: 1 in]
            }
            frame #1 {
              w157 = u32[] [68228136, 235670073, 4294967264, 4294967295, 4294967295, 511]  # Global Reg (default)
              w156 = u32 65535  # LayerID & ChipID
              # "default values to equalize"
              n33 = case shown="True" w153 {
                selector: w153 -> [w187 w189]
                tunnel: w156 -> [w188 w191]
                tunnel: [_ w197] -> w165
                tunnel: [_ w196] -> w164
                tunnel: [_ w195] -> w163
                tunnel: [_ w194] -> w146
                tunnel: [w186 w193] -> w162
                tunnel: w157 -> [_ w192]
                tunnel: [w188 w191] -> w160
                tunnel: w158 -> [_ w190]
                tunnel: [w187 w189] -> w159
                tunnel: w154 -> [w186 _]
                frame False {
                  # "Hardware 1 not enabled"
                }
                frame True {
                  # "Hardware 1 enabled"
                  n34 = call "OpenEthConnection.vi"("Port"=u16 80, "IP address"=w190) -> ("error out"=w203:errorcluster, "connection ID out"=w204:refnum<k5>)  [unwired: 7 in, 1 out]
                  n35 = call "Reset_FPGA_Module.vi"("error in (no error)"=w203, "connection ID"=w204) -> ("error out"=w200:errorcluster, "connection ID out"=w201:refnum<k5>, "Answer to Reset"=w195:string)  [unwired: 7 in]
                  n36 = call "ProgramGlobalReg.vi"("Global Reg"=w192, "error in (no error)"=w200, "ChipID"=w191, "LayerID"=w191, "connection ID"=w201) -> ("error out"=w196:errorcluster, "OK?"=w193:bool, "connection ID out"=w197:refnum<k5>, "Program done"=w199:string[])  [unwired: 2 in, 1 out]
                  n37 = Index Array "Index Array"(array=w199, index=1) -> (element=w194:string)
                }
              }
              n38 = case shown="True" w154 {
                selector: w154 -> [w169 w170]
                tunnel: w156 -> [_ w172]
                tunnel: [_ w178] -> w152
                tunnel: [_ w177] -> w151
                tunnel: [_ w176] -> w148
                tunnel: [_ w175] -> w147
                tunnel: [w168 w174] -> w149
                tunnel: w157 -> [_ w173]
                tunnel: w155 -> [_ w171]
                tunnel: [w169 w170] -> w150
                tunnel: w153 -> [w168 _]
                tunnel: w146 -> [_ _]
                frame False {
                  # "Hardware 2 not enabled"
                }
                frame True {
                  # "Hardware 2 enabled"
                  n39 = call "OpenEthConnection.vi"("Port"=u16 80, "IP address"=w171) -> ("error out"=w184:errorcluster, "connection ID out"=w185:refnum<k5>)  [unwired: 7 in, 1 out]
                  n40 = call "Reset_FPGA_Module.vi"("error in (no error)"=w184, "connection ID"=w185) -> ("error out"=w181:errorcluster, "connection ID out"=w182:refnum<k5>, "Answer to Reset"=w176:string)  [unwired: 7 in]
                  n41 = call "ProgramGlobalReg.vi"("Global Reg"=w173, "error in (no error)"=w181, "ChipID"=w172, "LayerID"=w172, "connection ID"=w182) -> ("error out"=w177:errorcluster, "OK?"=w174:bool, "connection ID out"=w178:refnum<k5>, "Program done"=w180:string[])  [unwired: 2 in, 1 out]
                  n42 = Index Array "Index Array"(array=w180, index=1) -> (element=w175:string)
                }
              }
              "Global Reg (hex)" <- w157
            }
            frame #2 {
              n43 = And(x=w211, y=w208) -> (x .and. y?=w207:bool)
              n44 = property on="Operation text" class="Str"(reference=w221, error in=w220, "Value"="Equalizing with HV...\nProgramming Pixel Regs...") -> ()  [unwired: 2 out]
            }
            frame #3 {
              w227 = "\r"
              n45 = call "EQ+px parameters.vi"() -> ("PixelReg (hex)"=w225:u32[], "I Leak out"=→"I Leak":u8, "EQ parameters (cluster) out"=w223:T4)  [unwired: 3 in]
              "PixelReg (hex)" <- w225
              n46 = local read "Chip ID list 1i2"() -> (w226:u32[])
              n47 = local write "EQ parameters (cluster)"(w223) -> ()
              n48 = case shown="True" w235 {
                tunnel: [_ w278] -> w248
                tunnel: [w266 w273] -> w233
                tunnel: w239 -> [_ w272]
                tunnel: w247 -> [_ w271]
                tunnel: w246 -> [w266 w270]
                tunnel: w225 -> [_ w269]
                tunnel: [w265 w268] -> w240
                tunnel: w236 -> [w265 _]
                tunnel: w226 -> [_ w267]
                frame False {
                  # "Hardware 1 not enabled"
                }
                frame True {
                  # "Hardware 1 enabled"
                  n49 = call "ProgramPixelReg.vi"("Chip ID list"=w267, "Pixel Register"=w269, "error in (no error)"=w270, "ChipID"=w272, "LayerID"=w272, "connection ID"=w271) -> ("error out"=w275:errorcluster, "OK?"=w268:bool, "connection ID out"=w274:refnum<k5>, "Program done"=w277:string[])  [unwired: 1 in, 1 out]
                  n50 = Index Array "Index Array"(array=w277, index=1) -> (element=w278:string)
                  n51 = call "CloseEthConnection.vi"("error in (no error)"=w275, "connection ID"=w274) -> ("error out"=w273:errorcluster)  [unwired: 9 in]
                }
              }
              n52 = case shown="True" w236 {
                tunnel: [_ w264] -> w230
                tunnel: [w252 w259] -> w232
                tunnel: w239 -> [_ w258]
                tunnel: w238 -> [_ w257]
                tunnel: w237 -> [w252 w256]
                tunnel: w225 -> [_ w255]
                tunnel: [w251 w254] -> w231
                tunnel: w235 -> [w251 _]
                tunnel: w226 -> [_ w253]
                frame False {
                  # "Hardware 2 not enabled"
                }
                frame True {
                  # "Hardware 2 enabled"
                  n53 = call "ProgramPixelReg.vi"("Chip ID list"=w253, "Pixel Register"=w255, "error in (no error)"=w256, "ChipID"=w258, "LayerID"=w258, "connection ID"=w257) -> ("error out"=w261:errorcluster, "OK?"=w254:bool, "connection ID out"=w260:refnum<k5>, "Program done"=w263:string[])  [unwired: 1 in, 1 out]
                  n54 = Index Array "Index Array"(array=w263, index=1) -> (element=w264:string)
                  n55 = call "CloseEthConnection.vi"("error in (no error)"=w261, "connection ID"=w260) -> ("error out"=w259:errorcluster)  [unwired: 9 in]
                }
              }
              n56 = Merge Errors(w233, w232) -> (w234:errorcluster)
              n57 = Unbundle By Name(w234) -> ("status"=w241:bool)
              n58 = call <vilib>:"Simple Error Handler.vi"("error in (no error)"=w234) -> ()  [unwired: 4 in, 5 out]
              n59 = Concatenate Strings "Concatenate Strings"(w245, w244, w248, w227, w227, w228, w229, w230) -> (w250:string)
              n60 = Compound Arithmetic op=AND(invert w241, w240, w243, w231) -> (w249:bool)
              n61 = property on="Error tick" class="Bool (strict)"(reference=w242, "Value"=w241) -> ()  [unwired: 1 in, 2 out]
              n62 = case shown="True" w249 {
                tunnel: w250 -> [_ w280]
                frame False {
                  # "error"
                }
                frame True {
                  # "OK x3"
                  n63 = call "MessageTimeOk.vi"("time (ms)"=3500, "missage"=w280) -> ()  [unwired: 4 in]
                }
              }
            }
          }
        }
        frame #2 {
          w283 = u32[][] [[0, 6], [7, 13], [14, 19], [20, 26], [27, 33], [34, 39], [40, 46], [47, 53], [54, 59], [60, 66], [67, 73], [74, 79], [80, 86], [87, 93], [94, 99]]  # steps of pixels
          w292 = 2028  # 2028xU32 per Layer
          # "Desactiva busy per permetre\nmesura de temperatura\ndurant EQ analisi i report viewer."
          # "row: all EQ DATA + Report (1 Layer)\ncol:  /elements U32 de la Layer/"
          # "Inicialitza\nall EQ DATA +REPORT\nrow: 1 Layer"
          # "2) EQUALITZACIÓ with HV"
          n64 = local read "quants Layer"() -> (w291:i32)
          n65 = disable-structure shown="Enabled" {
            disable-tunnel: [u32[][] [[0, 14], [15, 29], [30, 44], [45, 59], [60, 74], [75, 89], [90, 99]] ("steps of pixels") u32[][] [[0, 99]] ("steps of pixels")] -> w281
            frame Disabled {
              # "7 steps"
            }
            frame Enabled {
              # "1 step"
            }
          }
          n66 = Initialize Array(u32 0, w291, w292) -> (w309:u32[][])
          n67 = Select(t=w281, s=w284, f=w283) -> (s? t:f=w285:u32[][])
          n68 = for {
            tunnel: [w339] -> w294
            tunnel: w285 -> [w338] mode=indexing
            shift-right: [w336] -> w308
            shift-left: w309 -> [w337]
            tunnel: w307 -> [w334]
            tunnel: w306 -> [w335]
            tunnel: w305 -> [w333]
            tunnel: w304 -> [w332]
            tunnel: w303 -> [w331]
            tunnel: w302 -> [w330]
            tunnel: w301 -> [w329]
            tunnel: w300 -> [w328]
            tunnel: w299 -> [w327]
            tunnel: w298 -> [w326]
            tunnel: w297 -> [w325]
            tunnel: w296 -> [w324]
            tunnel: w295 -> [w323]
            tunnel: w293 -> [w322]
            tunnel: w290 -> [w321]
            tunnel: w289 -> [w320]
            tunnel: w288 -> [w319]
            tunnel: [w318] -> w286
            tunnel: "Stop subVI Refnum" -> [w313]
            i -> [w317]
            # "Sequencia d'equalitzacions parcials"
            n69 = Quotient & Remainder(x=w317, y=8) -> (x-y*floor(x/y)=w314:i32, floor(x/y)=w315:i32)
            n70 = stacked-sequence {
              seq-local: [_ _ _ w466 _ _ _] -> [_ _ _ _ _ w591 _]
              tunnel: [_ _ _ w483 _ _ _] -> w339
              tunnel: w338 -> [w355 w360 _ w494 _ _ _]
              tunnel: w337 -> [_ _ _ w471 _ _ _]
              tunnel: [_ _ _ w470 _ _ _] -> w336
              tunnel: w315 -> [w357 _ _ _ _ _ w654]
              tunnel: w335 -> [_ _ w416 _ _ _ _]
              tunnel: w334 -> [w352 _ _ _ _ _ _]
              tunnel: w333 -> [_ _ w417 _ _ _ _]
              tunnel: w332 -> [w349 _ w414 _ _ _ _]
              tunnel: w331 -> [_ _ _ _ _ _ _]
              tunnel: w330 -> [w348 _ _ _ _ _ _]
              tunnel: w329 -> [_ _ _ _ _ w600 _]
              tunnel: w328 -> [_ _ _ _ _ w601 _]
              tunnel: w327 -> [w347 _ _ _ _ w598 _]
              tunnel: w326 -> [w345 _ _ _ _ _ w653]
              tunnel: w325 -> [_ w368 _ _ w538 _ _]
              tunnel: w324 -> [_ w371 _ _ w536 _ _]
              tunnel: w323 -> [_ w367 _ w482 w540 _ _]
              tunnel: w322 -> [_ _ _ w489 _ _ _]
              tunnel: w321 -> [_ w362 w415 w469 w534 w599 _]
              tunnel: w320 -> [_ w364 w407 w460 w535 w588 w652]
              tunnel: w319 -> [_ _ w404 _ _ w585 _]
              tunnel: [_ _ _ _ _ _ w652] -> w318
              tunnel: w314 -> [w340 _ _ _ _ _ w651]
              tunnel: w313 -> [_ w359 _ _ w533 _ _]
              frame #0 {
                w346 = u8 0 ("ACQ-e2 barra")
                # "Inicialitzacions a la iteració"
                n71 = property on="EQ wHV steps barra" class="Arr (strict)"(reference=w345) -> (reference out=w343:refnum<vi>, error out=w342:errorcluster, "Value"=w344:u32[][])  [unwired: 1 in]
                n72 = Index Array "Index Array"(array=w355) -> (element #1=w354:u32, element #2=w353:u32)  [unwired: 2 in]
                n73 = in-place "In Place Element Structure" {
                  n74 = in-place-array #1(w344, w357, w340) -> ()  [unwired: 1 out]
                  n75 = in-place-array #1(u32 16756059) -> (w341:u32[][])  [unwired: 2 out]
                }
                n76 = Format Into String "Format Into String"(format string="Equalizing with HV...\nPixels from %d to %d ..." ("Value"), w354, w353) -> (resulting string=w351:string, error out=w350:errorcluster)  [unwired: 2 in]
                n77 = property on="Operation text" class="Str"(reference=w352, error in=w350, "Value"=w351) -> ()  [unwired: 2 out]
                n78 = property on="EQ wHV steps barra" class="Arr (strict)"(reference=w343, error in=w342, "Value"=w341) -> ()  [unwired: 2 out]
                n79 = property on="etapa2 barra" class="Slide (strict)"(reference=w349, "Value"=w346) -> ()  [unwired: 1 in, 2 out]
                n80 = property on="etapa3 barra" class="Slide (strict)"(reference=w348, "Value"=w346) -> ()  [unwired: 1 in, 2 out]
                n81 = property on="etapa5 barra" class="Slide (strict)"(reference=w347, "Value"=w346) -> ()  [unwired: 1 in, 2 out]
              }
              frame #1 {
                # "Etapa 1:  rampa pujada HV"
                n82 = flat-sequence {
                  tunnel: w371 -> [w383]
                  tunnel: [w383] -> w365
                  tunnel: w364 -> [w382]
                  tunnel: [w380] -> w363
                  tunnel: w362 -> [w380]
                  tunnel: [w379] -> w361
                  tunnel: w360 -> [w379]
                  tunnel: [w387] -> w374
                  tunnel: [w389] -> w370
                  tunnel: [w388] -> w369
                  tunnel: w365 -> [w391]
                  tunnel: w363 -> [w385]
                  tunnel: w361 -> [w384]
                  frame #0 {
                    # "Desactiva busy per permetre\nmesura de temperatura\ndurant rampa HV i temps H"
                    n83 = property on="busy = F" class="Bool (strict)"(reference=w382, "Value"=FALSE) -> ()  [unwired: 1 in, 2 out]
                  }
                  frame #1 {
                    n84 = while {
                      tunnel: w385 -> [w401]
                      tunnel: w384 -> [w403]
                      i -> [w397]
                      stop <- w394 stop-if-true
                      # "no cal en 1a\nEQ parcial"
                      # "temps màx\n10 s"
                      # "espera rebre permís"
                      n85 = Index Array "Index Array"(array=w403) -> (element=w402:u32)  [unwired: 1 in]
                      n86 = Wait on Notification(notifier=w401, timeout in ms (-1)=1000) -> (notification=w399:string)  [unwired: 2 in, 3 out]
                      n87 = Equal To 0?(x=w402) -> (x = 0?=w393:bool)
                      n88 = Equal?(x=w399, y="Start HV") -> (x = y?=w395:bool)
                      n89 = Greater?(x=w397, y=9) -> (0:w392:bool)
                      n90 = Compound Arithmetic op=OR "OR"(w393, w395, w392) -> (w394:bool)
                    }
                    n91 = local read "HV parameters"() -> (w387:T3)
                    n92 = property on="HV string" class="Str"(reference=w391, "Value"="HV ramping" ("HV String"), "Text.FontColor"=u32 15365376) -> (reference out=w389:refnum<vi>, error out=w388:errorcluster)  [unwired: 1 in]
                  }
                }
                n93 = call "HV_drive.vi"("Stop subVI Refnum"=w359, "HV level Refnum"=w368, "HV parameters"=w374) -> ("error out"=w373:errorcluster, "HV level (last value)"=w372:dbl)  [unwired: 1 in]
                n94 = flat-sequence {
                  tunnel: w372 -> [_]
                  tunnel: w370 -> [w377]
                  tunnel: w369 -> [w376]
                  frame #0 {
                    n95 = property on="HV string" class="Str"(reference=w377, error in=w376, "Value"="HV presence!" ("HV String"), "Text.FontColor"=u32 16711680) -> ()  [unwired: 2 out]
                  }
                }
                n96 = Unbundle By Name(w373) -> ("status"=w366:bool)
                n97 = call <vilib>:"Simple Error Handler.vi"("error in (no error)"=w373) -> ()  [unwired: 4 in, 5 out]
                n98 = property on="Error tick" class="Bool (strict)"(reference=w367, "Value"=w366) -> ()  [unwired: 1 in, 2 out]
              }
              frame #2 {
                # "Etapa 2:  temps inicial a HV_H"
                n99 = flat-sequence {
                  tunnel: w417 -> [w427]
                  tunnel: w416 -> [w424]
                  tunnel: w415 -> [w423]
                  tunnel: w414 -> [w420]
                  tunnel: [w428] -> w413
                  tunnel: [w425] -> w412
                  tunnel: [w424] -> w411
                  tunnel: [w420] -> w410
                  tunnel: [w419] -> w408
                  tunnel: w407 -> [w419]
                  tunnel: [w418] -> w405
                  tunnel: w404 -> [w418]
                  tunnel: w413 -> [w432]
                  tunnel: w412 -> [w433]
                  tunnel: w411 -> [w431]
                  tunnel: w410 -> [w434]
                  tunnel: [w430] -> w409
                  tunnel: w408 -> [w430]
                  tunnel: [w429] -> w406
                  tunnel: w405 -> [w429]
                  tunnel: w409 -> [w454]
                  tunnel: w406 -> [w453]
                  frame #0 {
                    # "Start Ileak measurement"
                    n100 = property on="etapa2 Actual time" class="DigNum (strict)"(reference=w427, "Value"=u32 0 ("ACQ-e2 Actual time")) -> (reference out=w425:refnum<vi>)  [unwired: 1 in, 1 out]
                    n101 = Send Notification(notification="Ileak ini+Start", notifier=w423) -> (error out=w422:errorcluster)  [unwired: 1 in, 1 out]
                    n102 = Tick Count (ms)() -> (millisecond timer value=w428:u32)
                    n103 = call <vilib>:"Simple Error Handler.vi"("error in (no error)"=w422) -> ()  [unwired: 4 in, 5 out]
                  }
                  frame #1 {
                    n104 = while {
                      tunnel: w432 -> [w450]
                      tunnel: w433 -> [w439]
                      tunnel: w431 -> [w438]
                      tunnel: w434 -> [w436]
                      stop <- w441 stop-if-true
                      n105 = property on="etapa2 Waiting time" class="DigNum (strict)"(reference=w438) -> ("Value"=w437:u32)  [unwired: 1 in, 2 out]
                      n106 = Tick Count (ms)() -> (millisecond timer value=w451:u32)
                      n107 = Subtract(x=w451, y=w450) -> (x-y=w449:u32)
                      n108 = Quotient & Remainder(x=w449, y=u32 1000) -> (floor(x/y)=w440:u32)  [unwired: 1 out]
                      n109 = Greater Or Equal?(x=w440, y=w437) -> (x >= y?=w441:bool)
                      n110 = To Double Precision Float(number=w440) -> (double precision float=w442:dbl)
                      n111 = To Double Precision Float(number=w437) -> (double precision float=w443:dbl)
                      n112 = property on="etapa2 Actual time" class="DigNum (strict)"(reference=w439, "Value"=w440) -> ()  [unwired: 1 in, 2 out]
                      n113 = Wait Until Next ms Multiple(millisecond multiple=u32 100) -> ()  [unwired: 1 out]
                      n114 = Divide(x=w442, y=w443) -> (x/y=w446:dbl)
                      n115 = Multiply(x=w446, y=100.0) -> (x*y=w444:dbl)
                      n116 = To Unsigned Byte Integer(number=w444) -> (unsigned 8bit integer=w435:u8)
                      n117 = property on="etapa2 barra" class="Slide (strict)"(reference=w436, "Value"=w435) -> ()  [unwired: 1 in, 2 out]
                    }
                  }
                  frame #2 {
                    # "Reactiva busy per procedir a l'equalització"
                    n118 = flat-sequence {
                      tunnel: w454 -> [w457]
                      tunnel: w453 -> [w455]
                      tunnel: [w455] -> w452
                      tunnel: w452 -> [w458]
                      frame #0 {
                        n119 = property on="busy = T" class="Bool (strict)"(reference=w457, "Value"=TRUE) -> ()  [unwired: 1 in, 2 out]
                      }
                      frame #1 {
                        n120 = Wait (ms)(milliseconds to wait=w458) -> ()  [unwired: 1 out]
                      }
                    }
                  }
                }
              }
              frame #3 {
                w485 = u32 65535  # LayerID & ChipID
                w488 = u32 1250000  # = 1/800n
                # "Endreça per Layer"
                # "row: all EQ DATA + Report (1 Layer)\ncol:  /elements U32 de la Layer/"
                # "First and Last Pixels"
                # "all EQ DATA + REPORT"
                # "Etapa 3:  equalització parcial"
                n121 = property on="busy = T" class="Bool (strict)"(reference=w460, "Value"=TRUE) -> (reference out=w459:refnum<vi>)  [unwired: 1 in, 1 out]
                n122 = Index Array "Index Array"(array=w494) -> (element #1=w490:u32, element #2=w468:u32)  [unwired: 2 in]
                n123 = flat-sequence {
                  tunnel: w482 -> [w503]
                  tunnel: [w503] -> w481
                  tunnel: [w502] -> w477
                  tunnel: w469 -> [w500]
                  tunnel: w459 -> [_]
                  tunnel: w492 -> [w511]
                  tunnel: w491 -> [w510]
                  tunnel: [w514] -> w474
                  tunnel: w481 -> [w516]
                  tunnel: [w507] -> w480
                  tunnel: [w506] -> w479
                  tunnel: [w516] -> w478
                  tunnel: w477 -> [w515]
                  tunnel: [w515] -> w476
                  tunnel: [w505] -> w464
                  tunnel: [w527] -> w475
                  tunnel: [w519] -> w483
                  tunnel: [w528] -> w493
                  tunnel: w480 -> [w528]
                  tunnel: w479 -> [w517]
                  tunnel: w478 -> [w527]
                  tunnel: w476 -> [w521]
                  tunnel: w466 -> [w522]
                  tunnel: [w520] -> w465
                  tunnel: w464 -> [w520]
                  tunnel: [w517] -> w462
                  frame #0 {
                    # "START Crono"
                    n124 = Send Notification(notification="EQcrono Start", notifier=w500) -> (notifier out=w502:refnum<notifier>, error out=w501:errorcluster)  [unwired: 1 in]
                    n125 = call <vilib>:"Simple Error Handler.vi"("error in (no error)"=w501) -> ()  [unwired: 4 in, 5 out]
                  }
                  frame #1 {
                    # "Equalization"
                    n126 = local read "Addresses Cluster"() -> (w513:T1)
                    n127 = local read "Global Reg (hex)"() -> (w509:u32[])
                    n128 = local read "PixelReg (hex)"() -> (w508:u32[])
                    n129 = call "subop_x2_Equalization.vi"("Addresses Cluster"=w513, "Equalization parameters"=w511, "Equalization timeout"=w510, "Global Reg (hex)"=w509, "PixelReg (hex)"=w508) -> ("EQ Data and Report"=w514:u32[], "timeout or error"=w506:bool, "answers done"=w505:string, "error out"=w512:errorcluster, "EQ timeout"=w507:bool)  [unwired: 10 in]
                    n130 = call <vilib>:"Simple Error Handler.vi"("error in (no error)"=w512) -> ()  [unwired: 4 in, 5 out]
                  }
                  frame #2 {
                    # "False: grava sempre"
                    # "ordenen també\n'Ileak Stop'"
                    # "STOP/EXIT Crono"
                    n131 = Select(t="EQcrono Exit", s=w522, f="EQcrono Stop") -> (s? t:f=w525:string)
                    n132 = And(x=FALSE, y=w517) -> (x .and. y?=w519:bool)
                    n133 = Send Notification(notification=w525, notifier=w521) -> (error out=w526:errorcluster)  [unwired: 1 in, 1 out]
                    n134 = call <vilib>:"Simple Error Handler.vi"("error in (no error)"=w526) -> ()  [unwired: 4 in, 5 out]
                  }
                }
                n135 = Bundle By Name(cluster="EQ parameters (cluster)", "First PIXEL"=w490, "Last PIXEL"=w468) -> (w487:T4)
                n136 = call "EQ_parameters_Edit.vi"("EQ parameters in"=w487) -> ("EQ parameters (hex)"=w492:u32[], "Number of pixels"=w473:u32)  [unwired: 4 in, 1 out]
                n137 = call "EQ_timeout_autocalcul.vi"("Number of pixels"=w473, "Chip ID"=w485, "Layer ID"=w485) -> ("EQ timeout auto (s)"=w484:u32)  [unwired: 8 in]
                n138 = Multiply(x=w484, y=w488) -> (x*y=w491:u32)
                n139 = property on="EQ timeout auto" class="DigNum (strict)"(reference=w489, "Value"=w484) -> ()  [unwired: 1 in, 2 out]
                n140 = local read "Chip ID list 1i2"() -> (w463:u32[])
                n141 = call "EQ_DATA_presort.vi"("EQ Data and Report"=w474, "number of pixels"=w473, "Chip ID list"=w463) -> ("Data+Report ordLayers"=w472:u32[][])  [unwired: 8 in]
                n142 = Equal?(x=w468, y=u32 99) -> (x = y?=w466:bool)
                n143 = for {
                  tunnel: w490 -> [w499]
                  tunnel: w468 -> [w498]
                  tunnel: w472 -> [w497] mode=indexing
                  tunnel: w471 -> [w496] mode=indexing
                  tunnel: [w495] -> w470 mode=indexing
                  # "indexat per Layer"
                  n144 = call "Merge EQ parcials.vi"("EQ DATA + REPORT (partial EQ)"=w497, "Last Pixel"=w498, "First Pixel"=w499, "all EQ DATA + REPORT in"=w496) -> ("all EQ DATA + REPORT out"=w495:u32[])  [unwired: 7 in]
                }
                n145 = property on="Error tick" class="Bool (strict)"(reference=w475, "Value"=w483) -> ()  [unwired: 1 in, 2 out]
                n146 = case shown="False" w462 {
                  tunnel: w465 -> [w529 _]
                  frame False {
                    # "if no error, Done message"
                    n147 = call "MessageTimeOk.vi"("time (ms)"=5200, "missage"=w529) -> ()  [unwired: 4 in]
                  }
                  frame True {
                  }
                }
                n148 = case shown="True" w493 {
                  frame False {
                  }
                  frame True {
                    n149 = call "MessageTimeOk.vi"("time (ms)"=5200, "missage"="Equalization timeout." ("message")) -> ()  [unwired: 4 in]
                  }
                }
              }
              frame #4 {
                # "Etapa 4:  rampa bajada HV"
                n150 = flat-sequence {
                  tunnel: [w549] -> w541
                  tunnel: w540 -> [w549]
                  tunnel: [w548] -> w539
                  tunnel: w538 -> [w548]
                  tunnel: [w547] -> w537
                  tunnel: w536 -> [w547]
                  tunnel: w535 -> [w545]
                  tunnel: w534 -> [w544]
                  frame #0 {
                    # "Desactiva busy per permetre\nmesura de temperatura\ndurant rampa HV i temps L"
                    n151 = while {
                      tunnel: w544 -> [w558]
                      i -> [w554]
                      stop <- w552 stop-if-true
                      # "temps màx\n10 s"
                      # "espera rebre permís"
                      n152 = Wait on Notification(notifier=w558, timeout in ms (-1)=1000) -> (notification=w556:string)  [unwired: 2 in, 3 out]
                      n153 = Equal?(x=w556, y="Start HV") -> (x = y?=w551:bool)
                      n154 = Greater?(x=w554, y=9) -> (0:w550:bool)
                      n155 = Or(x=w551, y=w550) -> (x .or. y?=w552:bool)
                    }
                    n156 = property on="busy = F" class="Bool (strict)"(reference=w545, "Value"=FALSE) -> ()  [unwired: 1 in, 2 out]
                  }
                }
                n157 = property on="HV level" class="Slide (strict)"(reference=w539) -> ("Value"=w542:dbl)  [unwired: 1 in, 2 out]
                n158 = Not Equal To 0?(x=w542) -> (x != 0?=w543:bool)
                n159 = case shown="True" w543 {
                  tunnel: w539 -> [_ w562]
                  tunnel: w537 -> [_ w561]
                  tunnel: w541 -> [_ w560]
                  tunnel: w533 -> [_ w559]
                  frame False {
                    # "HV = 0,   no cal baixada"
                  }
                  frame True {
                    n160 = flat-sequence {
                      tunnel: [w580] -> w563
                      tunnel: w561 -> [w584]
                      tunnel: [w582] -> w566
                      tunnel: [w581] -> w567
                      frame #0 {
                        n161 = local read "HV parameters"() -> (w580:T3)
                        n162 = property on="HV string" class="Str"(reference=w584, "Value"="HV ramping" ("HV String"), "Text.FontColor"=u32 15365376) -> (reference out=w582:refnum<vi>, error out=w581:errorcluster)  [unwired: 1 in]
                      }
                    }
                    n163 = call "HV_drive.vi"("Stop subVI Refnum"=w559, "HV level Refnum"=w562, "HV parameters"=w563) -> ("error out"=w564:errorcluster, "HV level (last value)"=w565:dbl)  [unwired: 1 in]
                    n164 = flat-sequence {
                      tunnel: w565 -> [w571]
                      tunnel: w566 -> [w578]
                      tunnel: w567 -> [w577]
                      frame #0 {
                        n165 = Equal To 0?(x=w571) -> (x = 0?=w576:bool)
                        n166 = Select(t="HV off", s=w576, f="HV presence!") -> (s? t:f=w570:string)
                        n167 = Select(t=u32 42533, s=w576, f=u32 16711680) -> (s? t:f=w569:u32)
                        n168 = property on="HV string" class="Str"(reference=w578, error in=w577, "Value"=w570, "Text.FontColor"=w569) -> ()  [unwired: 2 out]
                      }
                    }
                    n169 = Unbundle By Name(w564) -> ("status"=w568:bool)
                    n170 = call <vilib>:"Simple Error Handler.vi"("error in (no error)"=w564) -> ()  [unwired: 4 in, 5 out]
                    n171 = property on="Error tick" class="Bool (strict)"(reference=w560, "Value"=w568) -> ()  [unwired: 1 in, 2 out]
                  }
                }
              }
              frame #5 {
                # "Etapa 5:  temps final a HV_L"
                n172 = flat-sequence {
                  tunnel: w601 -> [w612]
                  tunnel: w600 -> [w608]
                  tunnel: w599 -> [w607]
                  tunnel: w598 -> [w604]
                  tunnel: [w613] -> w597
                  tunnel: [w610] -> w596
                  tunnel: [w608] -> w595
                  tunnel: [w605] -> w594
                  tunnel: [w604] -> w593
                  tunnel: [w603] -> w589
                  tunnel: w588 -> [w603]
                  tunnel: [w602] -> w586
                  tunnel: w585 -> [w602]
                  tunnel: w597 -> [w618]
                  tunnel: w596 -> [w617]
                  tunnel: w595 -> [w619]
                  tunnel: w594 -> [w620]
                  tunnel: w593 -> [w616]
                  tunnel: [w620] -> w592
                  tunnel: [w615] -> w590
                  tunnel: w589 -> [w615]
                  tunnel: [w614] -> w587
                  tunnel: w586 -> [w614]
                  tunnel: w592 -> [w645]
                  tunnel: w591 -> [w642]
                  tunnel: w590 -> [w639]
                  tunnel: w587 -> [w638]
                  frame #0 {
                    # "Start Ileak measurement"
                    n173 = property on="etapa5 Actual time" class="DigNum (strict)"(reference=w612, "Value"=u32 0 ("ACQ-e2 Actual time")) -> (reference out=w610:refnum<vi>)  [unwired: 1 in, 1 out]
                    n174 = Send Notification(notification="Ileak ini+Start", notifier=w607) -> (notifier out=w605:refnum<notifier>, error out=w606:errorcluster)  [unwired: 1 in]
                    n175 = Tick Count (ms)() -> (millisecond timer value=w613:u32)
                    n176 = call <vilib>:"Simple Error Handler.vi"("error in (no error)"=w606) -> ()  [unwired: 4 in, 5 out]
                  }
                  frame #1 {
                    n177 = while {
                      tunnel: w618 -> [w636]
                      tunnel: w617 -> [w625]
                      tunnel: w619 -> [w624]
                      tunnel: w616 -> [w622]
                      stop <- w627 stop-if-true
                      # "et5: temps final a HV_L"
                      n178 = property on="etapa5 Waiting time" class="DigNum (strict)"(reference=w624) -> ("Value"=w623:u32)  [unwired: 1 in, 2 out]
                      n179 = Tick Count (ms)() -> (millisecond timer value=w637:u32)
                      n180 = Subtract(x=w637, y=w636) -> (x-y=w635:u32)
                      n181 = Quotient & Remainder(x=w635, y=u32 1000) -> (floor(x/y)=w626:u32)  [unwired: 1 out]
                      n182 = Greater Or Equal?(x=w626, y=w623) -> (x >= y?=w627:bool)
                      n183 = To Double Precision Float(number=w626) -> (double precision float=w628:dbl)
                      n184 = To Double Precision Float(number=w623) -> (double precision float=w629:dbl)
                      n185 = property on="etapa5 Actual time" class="DigNum (strict)"(reference=w625, "Value"=w626) -> ()  [unwired: 1 in, 2 out]
                      n186 = Wait Until Next ms Multiple(millisecond multiple=u32 100) -> ()  [unwired: 1 out]
                      n187 = Divide(x=w628, y=w629) -> (x/y=w632:dbl)
                      n188 = Multiply(x=w632, y=100.0) -> (x*y=w630:dbl)
                      n189 = To Unsigned Byte Integer(number=w630) -> (unsigned 8bit integer=w621:u8)
                      n190 = property on="etapa5 barra" class="Slide (strict)"(reference=w622, "Value"=w621) -> ()  [unwired: 1 in, 2 out]
                    }
                  }
                  frame #2 {
                    # "Reactiva busy per seguir amb la seqüència"
                    # "Stop/Exit Ileak measurement"
                    n191 = flat-sequence {
                      tunnel: w639 -> [w649]
                      tunnel: w638 -> [w647]
                      tunnel: [w647] -> w640
                      tunnel: w640 -> [w650]
                      frame #0 {
                        n192 = property on="busy = T" class="Bool (strict)"(reference=w649, "Value"=TRUE) -> ()  [unwired: 1 in, 2 out]
                      }
                      frame #1 {
                        n193 = Wait (ms)(milliseconds to wait=w650) -> ()  [unwired: 1 out]
                      }
                    }
                    n194 = Select(t="Ileak Exit" ("notification"), s=w642, f="Ileak Stop" ("notification")) -> (s? t:f=w641:string)
                    n195 = Send Notification(notification=w641, notifier=w645) -> (error out=w646:errorcluster)  [unwired: 1 in, 1 out]
                    n196 = call <vilib>:"Simple Error Handler.vi"("error in (no error)"=w646) -> ()  [unwired: 4 in, 5 out]
                  }
                }
              }
              frame #6 {
                # "Finalització parcial"
                n197 = property on="EQ wHV steps barra" class="Arr (strict)"(reference=w653) -> (reference out=w657:refnum<vi>, error out=w656:errorcluster, "Value"=w658:u32[][])  [unwired: 1 in]
                n198 = in-place "In Place Element Structure" {
                  n199 = in-place-array #2(w658, w654, w651) -> ()  [unwired: 1 out]
                  n200 = in-place-array #2(u32 46120) -> (w655:u32[][])  [unwired: 2 out]
                }
                n201 = property on="EQ wHV steps barra" class="Arr (strict)"(reference=w657, error in=w656, "Value"=w655) -> ()  [unwired: 2 out]
              }
            }
          }
          n202 = property on="busy = F" class="Bool (strict)"(reference=w286, "Value"=FALSE) -> ()  [unwired: 1 in, 2 out]
        }
        frame #3 {
          # "Notify to thread Ileak measurement\nSend EQ report folder path"
          # "row: all EQ DATA + Report (1 Layer)\ncol:  /elements U32 de la Layer/"
          # "3) ANÀLISIS, save files"
          n203 = case shown="False" w668 {
            tunnel: w667 -> [w684 _]
            tunnel: w666 -> [w683 _]
            tunnel: [w673 _] -> w660
            tunnel: [w672 _] -> w665
            tunnel: [w671 _] -> w664
            frame False {
              # "No hi ha error: analitza i grava arxius"
              n204 = flat-sequence {
                tunnel: w684 -> [w694]
                tunnel: w683 -> [w693]
                tunnel: [w694] -> w682
                tunnel: [w691] -> w679
                tunnel: [w690] -> w677
                tunnel: [w686] -> w670
                tunnel: [w685] -> w669
                tunnel: w682 -> [w697]
                tunnel: [w701] -> w681
                tunnel: [w700] -> w680
                tunnel: w679 -> [w700]
                tunnel: [w699] -> w678
                tunnel: w677 -> [w699]
                tunnel: [w698] -> w674
                tunnel: w670 -> [w696]
                tunnel: w669 -> [w695]
                tunnel: w681 -> [w712]
                tunnel: w680 -> [w714]
                tunnel: w678 -> [w713]
                tunnel: [w712] -> w676
                tunnel: [w711] -> w675
                tunnel: w674 -> [w711]
                tunnel: w676 -> [w727]
                tunnel: w675 -> [w719]
                tunnel: [w720] -> w673
                tunnel: [w719] -> w672
                tunnel: [w718] -> w671
                frame #0 {
                  # "row: all EQ DATA + Report (1 Layer)\ncol:  /elements U32 de la Layer/"
                  # "Operation text"
                  n205 = local read "EQ parameters (cluster)"() -> (w689:T4)
                  n206 = Unbundle By Name(w689) -> ("TOT"=w688:u32, "ADC target"=w687:u32)
                  n207 = property on="Operation text" class="Str"(reference=w693, "Value"="Equalizing with HV...\nAnalyzing data...") -> (reference out=w691:refnum<vi>, error out=w690:errorcluster)  [unwired: 1 in]
                  n208 = To Unsigned Word Integer(number=w688) -> (unsigned 16bit integer=w686:u16)
                  n209 = To Unsigned Word Integer(number=w687) -> (unsigned 16bit integer=w685:u16)
                }
                frame #1 {
                  # "EQ DATA analysis"
                  n210 = for {
                    shift-right: [w707] -> w701
                    shift-left: w697 -> [w709]
                    tunnel: [w705] -> w698 mode=concatenating
                    tunnel: w697 -> [_] mode=indexing
                    tunnel: w696 -> [w704]
                    tunnel: w695 -> [w703]
                    i -> [w708]
                    w710 = u32 100  # number of pixels
                    # "indexat per Layers\n(manté ordre de ChipID list)"
                    n211 = Index Array "Index Array"(array=w709, index (row)=w708) -> (element=w702:u32[])  [unwired: 1 in]
                    n212 = call "EQ analysis.vi"("number of pixels"=w710, "TOT (us)"=w704, "ADC target"=w703, "EQ Data and Report"=w702) -> ("EQ Data and Report, analyzed"=w706:u32[], "quants pixels bons per Chip"=w705:u8[])  [unwired: 10 in]
                    n213 = Replace Array Subset "Replace Array Subset"(array=w709, new element=w706, index (row)=w708) -> (w707:u32[][])  [unwired: 1 in]
                  }
                }
                frame #2 {
                  # "Operation text"
                  n214 = property on="Operation text" class="Str"(reference=w714, error in=w713, "Value"="Equalizing with HV...\nSaving files...") -> ()  [unwired: 2 out]
                }
                frame #3 {
                  w716 = TRUE  # HV enabled
                  w732 = u8 0 items=["Equalization", "Acquisition"] ("Operation text")
                  # "Arxiu resum de\npixels bons per ChipID"
                  # "Grava EQ_DATA+REPORT per Chip\nInclou Grava_EQ_registers_u\nInclou Grava_EQ_report_u"
                  # "Arxiu conjunt tot EQ_DATA+REPORT"
                  # "Reshape all Layers EQ_DATA+REPORT"
                  # "Crea EQ folder path"
                  # "Save files"
                  n215 = local read "HV parameters"() -> (w733:T3)
                  n216 = Array Size(array=w727) -> (size(s)=w731:i32[])
                  n217 = Index Array "Index Array"(array=w731) -> (element #1=w729:i32, element #2=w730:i32)  [unwired: 2 in]
                  n218 = local read "I Leak"() -> (w735:u8)
                  n219 = Multiply(x=w729, y=w730) -> (x*y=w728:i32)
                  n220 = Unbundle By Name(w733) -> ("Final value"=w734:i16)
                  n221 = Reshape Array "Reshape Array"(w727, w728) -> (w725:u32[])
                  n222 = call "Path format.vi"("Operation type"=w732, "HV level"=w734, "I leakage"=w735, "HV enable button"=w716) -> ("folder path"=w720:path)  [unwired: 1 in]
                  n223 = call "EQ make summary.vi"("quants pixels bons per Chip"=w719) -> ("summary EQ"=w718:string)  [unwired: 4 in]
                  n224 = local write "Folder path: equalization reports"(w720) -> ()
                  n225 = local read "Chip ID list 1i2"() -> (w721:u32[])
                  n226 = call "Grava_EQ_u.vi"("all Layers EQ_DATA+REPORT"=w725, "number of pixels"=u32 100, "Folder path: equalization"=w720) -> ("subfolder path: text reports"=w723:path)  [unwired: 2 in]
                  n227 = call "Grava_summaryEQ.vi"("summary EQ"=w718, "quants pixels bons per Chip"=w719, "ChipID list"=w721, "file name"="EQ summary.txt", "subfolder path: text reports"=w723) -> ()  [unwired: 2 in]
                  n228 = call "Grava_ArrayInFile_int.vi"("format (%08x)"="%08x", "Array to save"=w725, "file name"="Equalization_Module_DATA.txt", "folder path"=w720) -> ()  [unwired: 1 in]
                }
              }
            }
            frame True {
              # "EQ timeout or error"
            }
          }
          n229 = Path To String(path=w660) -> (string=w661:string)
          n230 = Send Notification(notification=w661, notifier=w662) -> (error out=w663:errorcluster)  [unwired: 1 in, 1 out]
          n231 = call <vilib>:"Simple Error Handler.vi"("error in (no error)"=w663) -> ()  [unwired: 4 in, 5 out]
        }
        frame #4 {
          # "3) Open EQ Report Viewer with data"
          n232 = case shown="False" w741 {
            tunnel: w740 -> [w748 _]
            tunnel: w739 -> [w746 _]
            tunnel: w738 -> [w744 _]
            tunnel: w737 -> [w750 _]
            tunnel: w736 -> [w742 _]
            frame False {
              # "Show EQ summary window and EQ_report_viewer x4"
              n233 = flat-sequence {
                tunnel: w750 -> [w756]
                tunnel: [w754] -> w749
                tunnel: w748 -> [w754]
                tunnel: [w753] -> w747
                tunnel: w746 -> [w753]
                tunnel: [w752] -> w745
                tunnel: w744 -> [w752]
                tunnel: [w751] -> w743
                tunnel: w742 -> [w751]
                tunnel: w749 -> [w760]
                tunnel: w747 -> [w758]
                tunnel: w745 -> [w757]
                tunnel: w743 -> [w759]
                frame #0 {
                  n234 = property on="Operation text" class="Str"(reference=w756, "Value"="EQ report viewer open.") -> ()  [unwired: 1 in, 2 out]
                }
                frame #1 {
                  n235 = local read "Chip ID list 1i2"() -> (w761:u32[])
                  n236 = call "EQ choose report.vi"("Chip ID list"=w761, "quants pixels bons per Chip"=w760, "Folder path: EQ reports"=w759, "summary IDs"=w758, "summary EQ"=w757) -> ()  [unwired: 11 in]
                }
              }
            }
            frame True {
              # "EQ timeout or error"
            }
          }
        }
      }
    }
    frame True {
      # "connection not working"
      n237 = property on="Error tick" class="Bool (strict)"(reference=w762, "Value"=w763) -> ()  [unwired: 1 in, 2 out]
      n238 = One Button Dialog(message="The connection is NOT WORKING.\n\nCheck the wiring connection and the IP address.") -> ()  [unwired: 1 in, 1 out]
    }
  }
  "Folder path: equalization reports" <- w7
  "IDs summary" <- w6
  "EQ summary" <- w5
